vi "cDAQ_VI_Leo_Autotuning.vi"() -> ()   [LabVIEW 2022 SP3]
uses:
  <vilib>/addons/control/pid/autopid.llb/PID autotuning parameters.ctl
  <vilib>/Analysis/baseanly.llb/Mean (DBL).vi
  <vilib>/DAQmx/read.llb/DAQmx Read (Analog 1D Wfm NChan NSamp).vi
  STOP_GLOBAL.vi
  <vilib>/DAQmx/configure/timing.llb/DAQmx Timing (Sample Clock).vi
  <vilib>/addons/control/pid/pid.llb/PID Lead-Lag (DBL).vi
  <vilib>/addons/control/pid/pid.llb/PID Gain Schedule (DBL).vi
  <vilib>/addons/control/pid/pid.llb/PID (DBL).vi
  <vilib>/DAQmx/miscellaneous.llb/DAQmx Fill In Error Info.vi
  <vilib>/Analysis/NI_AALBase.lvlib
  <vilib>/addons/control/pid/NI_PID_pid.lvlib
  <vilib>/ptbypt/NI_PtbyPt.lvlib
  <resource>/objmgr/daqmx.rc
panel:
  out "Inlet Pressure":dynamicdata(graph)
  in  "Channel Array":dbl[](array[slide]) scale=0.0..5.067
  in  "Pressure Scheduling":T1(array[cluster])=[{"PID gains"={"Kc"=7.0, "Ti"=0.001, "Td"=0.0}, "max value"=0.0}] {"max value" format="%.2f"; "PID gains"."Td" format="%#.3g"; "PID gains"."Ti" format="%#.3g"; "PID gains"."Kc" format="%#.3g"}
  out "Runtime Passed?":bool
  in  "RunTime":dbl
  out "Entire Runtime":dbl
  out "Actual Clock Rate":dbl
  out "error out 4":errorcluster
  out "Setpoint profile":dbl
  out "Second Pressure Transducer":cluster{dbl[], dbl[]}(graph)
  out "Line Pressure":dynamicdata(graph)
  out "Servo Voltage Output":cluster{dbl[], dbl[]}(graph)
  in  "Tab Control":T2(tab)
  out "error out 5":errorcluster
  in  "stop":bool
  in  "Needle Valve Control":dbl[](array[slide]) scale=0.0..1.0
  out "Waveform Chart":cluster{"SP":dbl, dbl}(graph)
  out "Output":dbl(slide) scale=0.0..5.067
  out "Process Variable vs Setpoint":cluster{dbl[], dbl[]}[](graph)
  out "error out":errorcluster
  out "element":dbl
  out "MVT Process variable":dbl
  out "MVT Setpoint":dbl
  in  "SP":dbl format="%.2f"
  out "PID gains out":T3={"proportional gain (Kc)"=1.0, "integral time (Ti, min)"=0.01, "derivative time (Td, min)"=0.0} {"derivative time (Td, min)" format="%.3f"; "integral time (Ti, min)" format="%.3f"; "proportional gain (Kc)" format="%.3f"}
  in  "Insert Gain":bool
  out "output":dbl format="%.2f"
  in  "Autotune":bool
  in  "Reinitialize":bool
  in  "Automatic":bool=TRUE
  in  "Replace Gain":bool
  in  "alpha":dbl=nan format="%.2f"
  out "tuned PID gains":T3={"proportional gain (Kc)"=1.0, "integral time (Ti, min)"=0.01, "derivative time (Td, min)"=0.0} {"derivative time (Td, min)" format="%.3f"; "integral time (Ti, min)" format="%.3f"; "proportional gain (Kc)" format="%.3f"}
  out "Voltage Output":dynamicdata(graph)
  in  "autotuning parameters":T4={"type of controller"=0, "relay cycles"=3, "relay amplitude"=1.0, "control specifications"=2, "PV noise level"=0.1} {"PV noise level" format="%.2f"; "control specifications" items=["normal", "fast", "slow"]; "relay amplitude" format="%.2f"; "type of controller" items=["P", "PI", "PID"]}
  out "index out":i32
  in  "MV:":dbl(slide)=30.8641975308642 scale=0.0..5.067 scale format="%.1f"
  out "Waiting \nfor Start":bool=TRUE
  in  "Start VI":bool
  out "Time":dbl
  in  "Gain Schedule":T1(array[cluster])=[{"PID gains"={"Kc"=7.0, "Ti"=0.001, "Td"=0.0}, "max value"=0.0}] {"max value" format="%.2f"; "PID gains"."Td" format="%#.3g"; "PID gains"."Ti" format="%#.3g"; "PID gains"."Kc" format="%#.3g"}
  out "Steps on Servo":dbl[](array[numeric])
  out "Elapsed Time (s) 2":dbl caption="Elapsed Time (s)"
  out "HAS 3 SECONDS PASSED?":bool
  in  "PRESS TO START":bool
  out "All Channel Graph":cluster{dbl[], dbl[]}[](graph)
  out "Thrust":cluster{dbl[], dbl[]}(graph)
  out "Chamber Pressure":cluster{dbl[], dbl[]}(graph)
  out "Supply Pressure":cluster{dbl[], dbl[]}(graph)
  out "MassFlow":cluster{dbl[], dbl[]}(graph)
  out "Temperature":cluster{dbl[], dbl[]}(graph)
  out "error out 3":errorcluster caption="error out"
  out "error out 2":errorcluster
  in  "rate":dbl=1000.0 format="%0.2f"
  in  "number of samples":i32=100
  in  "File Format":string
  in  "File Name Out":string
  in  "Data Collection Folder":path
  out "Temperature":dynamicdata(graph)
  out "Thrust lb":dynamicdata(graph)
  in  "Types of Testing":enum32{"Test Firing", "Cold Flow Rig"}(tab)
  out "Saving Data":bool
  out "Filename Out":path
  in  "Collect Data?":bool=TRUE caption="Enable"
  in  "Collect Data? 2":bool=TRUE caption="Enable"
  out "Saving Data":bool
  out "Filename Out":path
  out "Supply Pressure PSI":dynamicdata(graph)
  out "Vol Flow L/min":dynamicdata(graph)
  out "Chamber Pressure PSI":dynamicdata(graph)
  # "DATA LOGGING INFORMATION"
  # "Control Loop"
  # "ANALOG VOLTAGE OUTPUT"
  # "RESULTS"
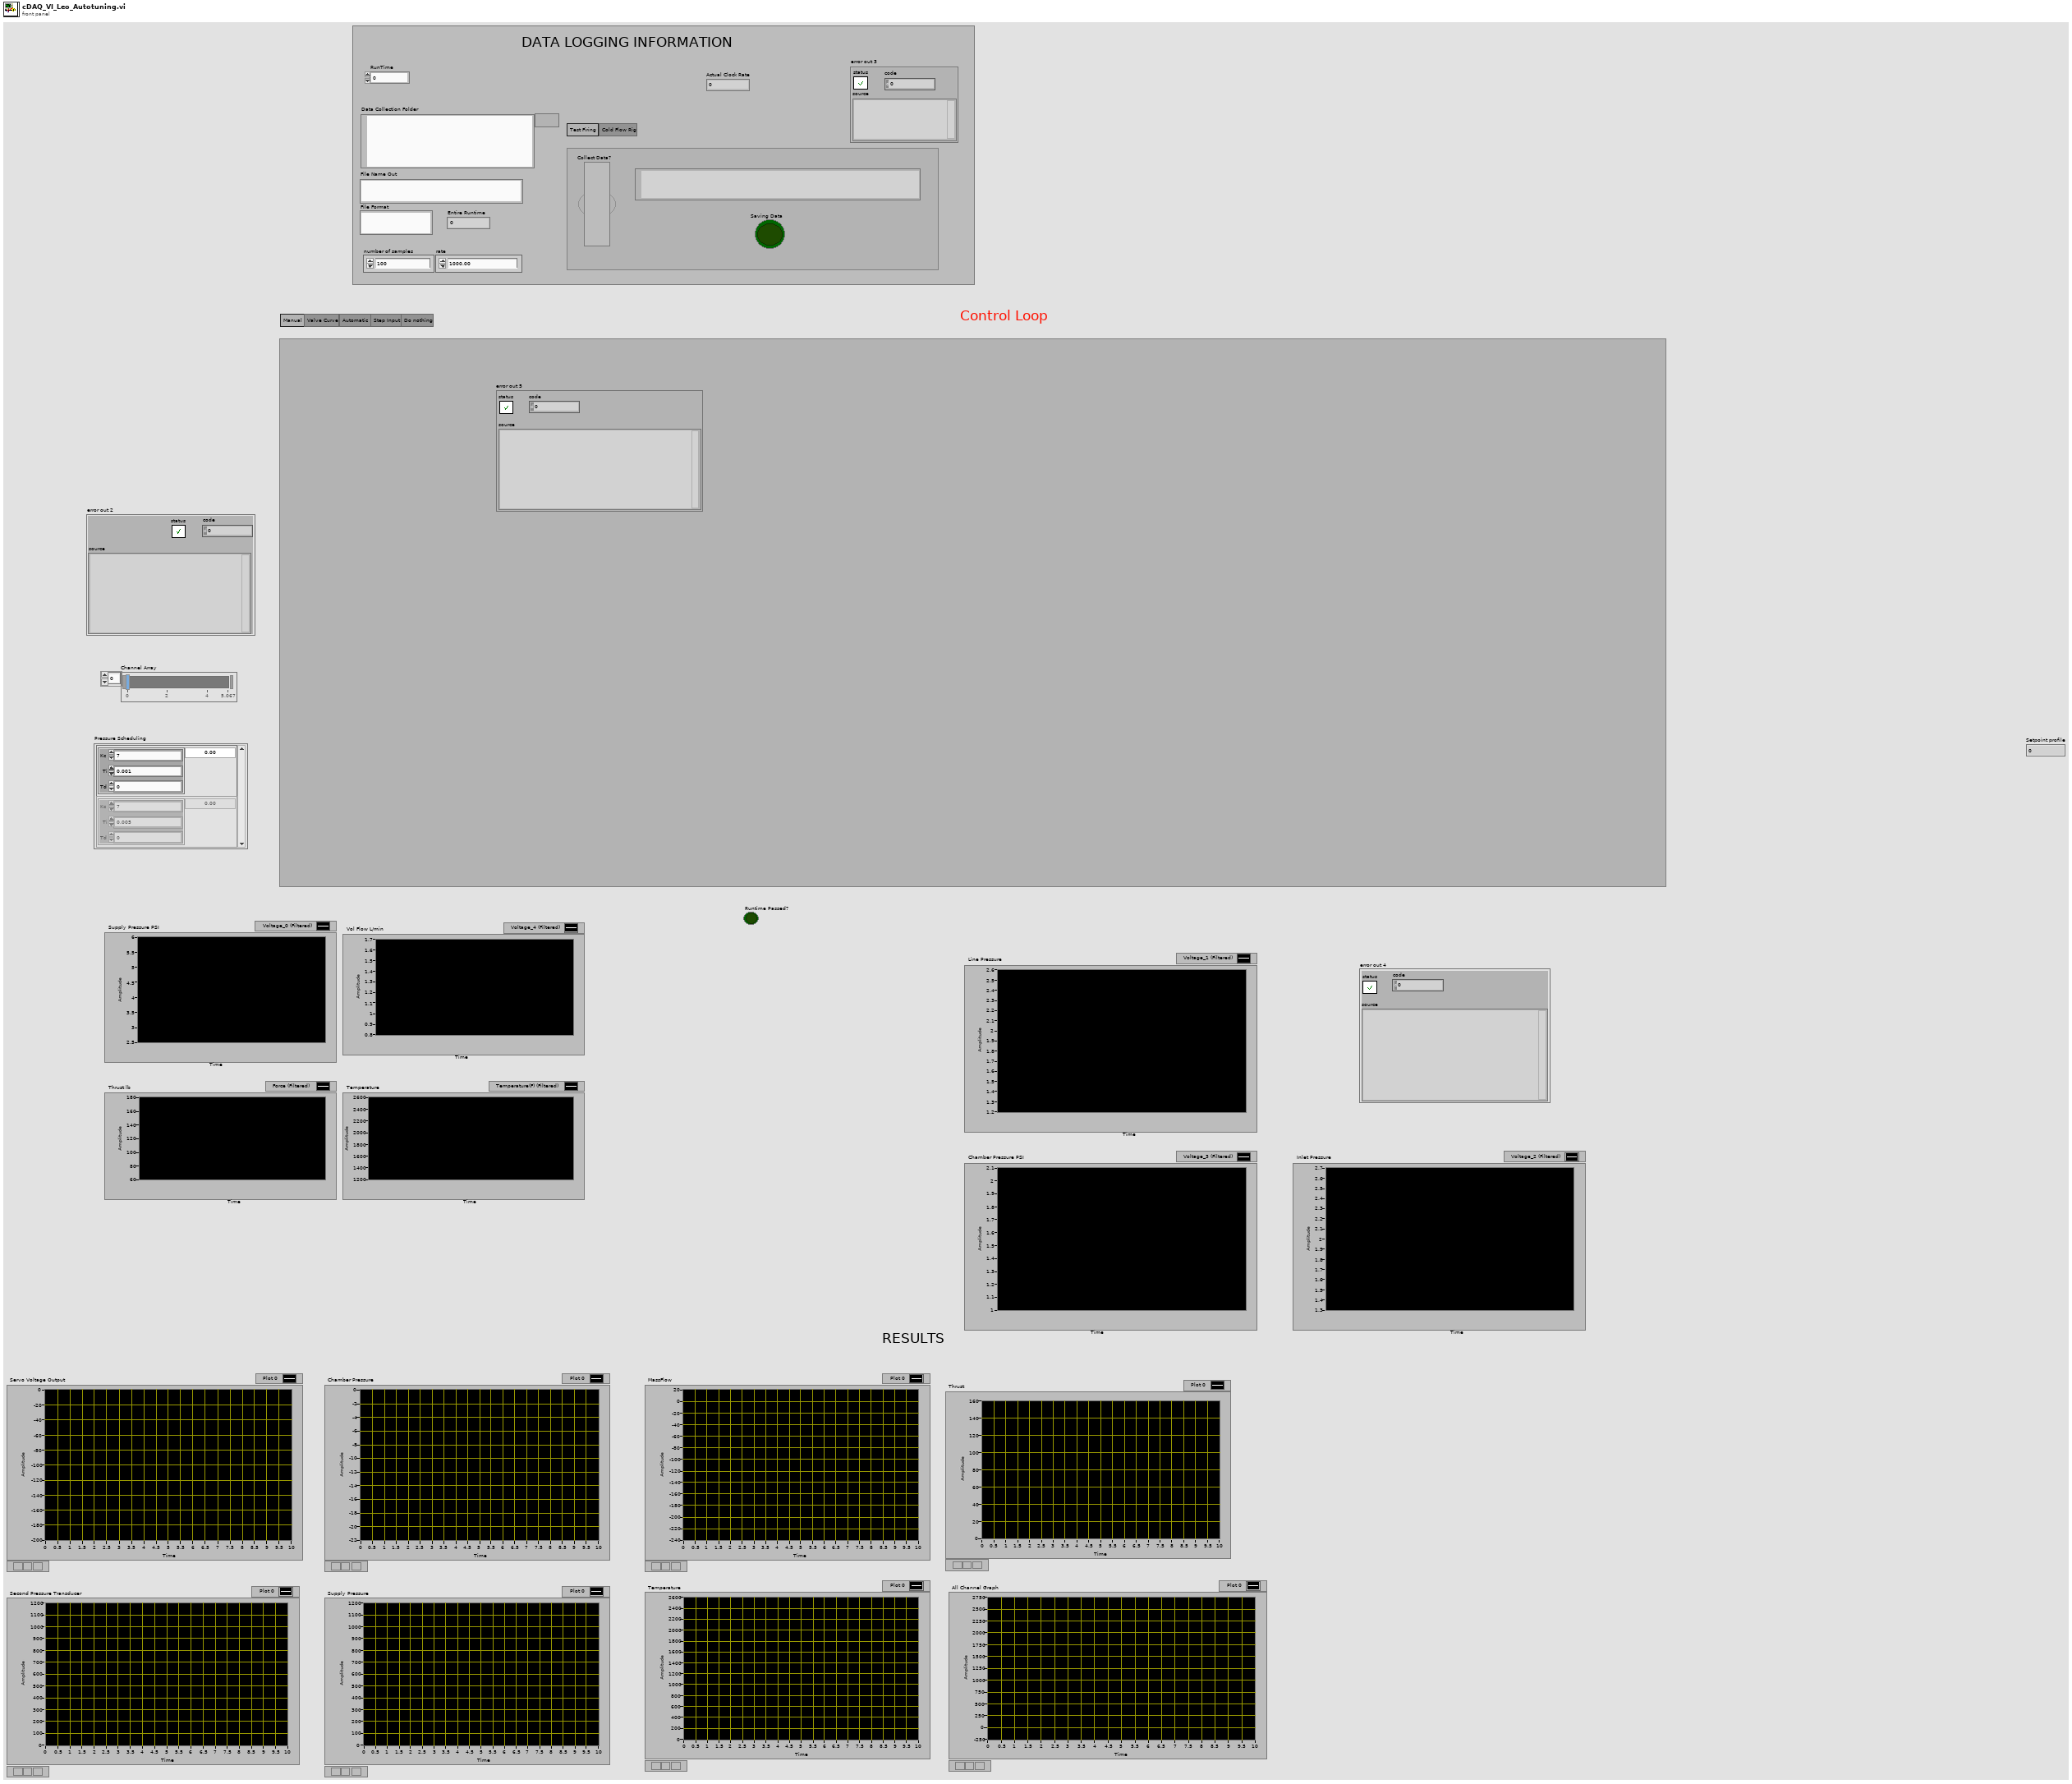
[diagram p1: front panel]
types:
  T1 = cluster{"PID gains":cluster{"Kc":dbl, "Ti":dbl, "Td":dbl}, "max value":dbl}[]
  T2 = enum32{"Manual", "Valve Curve", "Automatic", "Step Input", "Do nothing"}
  T3 = cluster{"proportional gain (Kc)":dbl, "integral time (Ti, min)":dbl, "derivative time (Td, min)":dbl}
  T4 = typedef "PID autotuning parameters.ctl" = cluster{"type of controller":u16, "relay cycles":i32, "relay amplitude":dbl, "control specifications":u16, "PV noise level":dbl}
  T5 = cluster{"Modulus":dbl, "Number of\nComplete Cycles":dbl}
  T6 = cluster{"PID gains":cluster{"Kc":dbl, "Ti":dbl, "Td":dbl}, "max value":dbl}
  T7 = cluster{"Tuned PID gains":cluster{"proportional gain (Kc)":dbl, "integral time (Ti, min)":dbl, "derivative time (Td, min)":dbl}, "MVT Process Variable":dbl}
  T8 = cluster{"Tuned PID gains":cluster{"proportional gain (Kc)":dbl, "integral time (Ti, min)":dbl, "derivative time (Td, min)":dbl}, "max value":dbl}
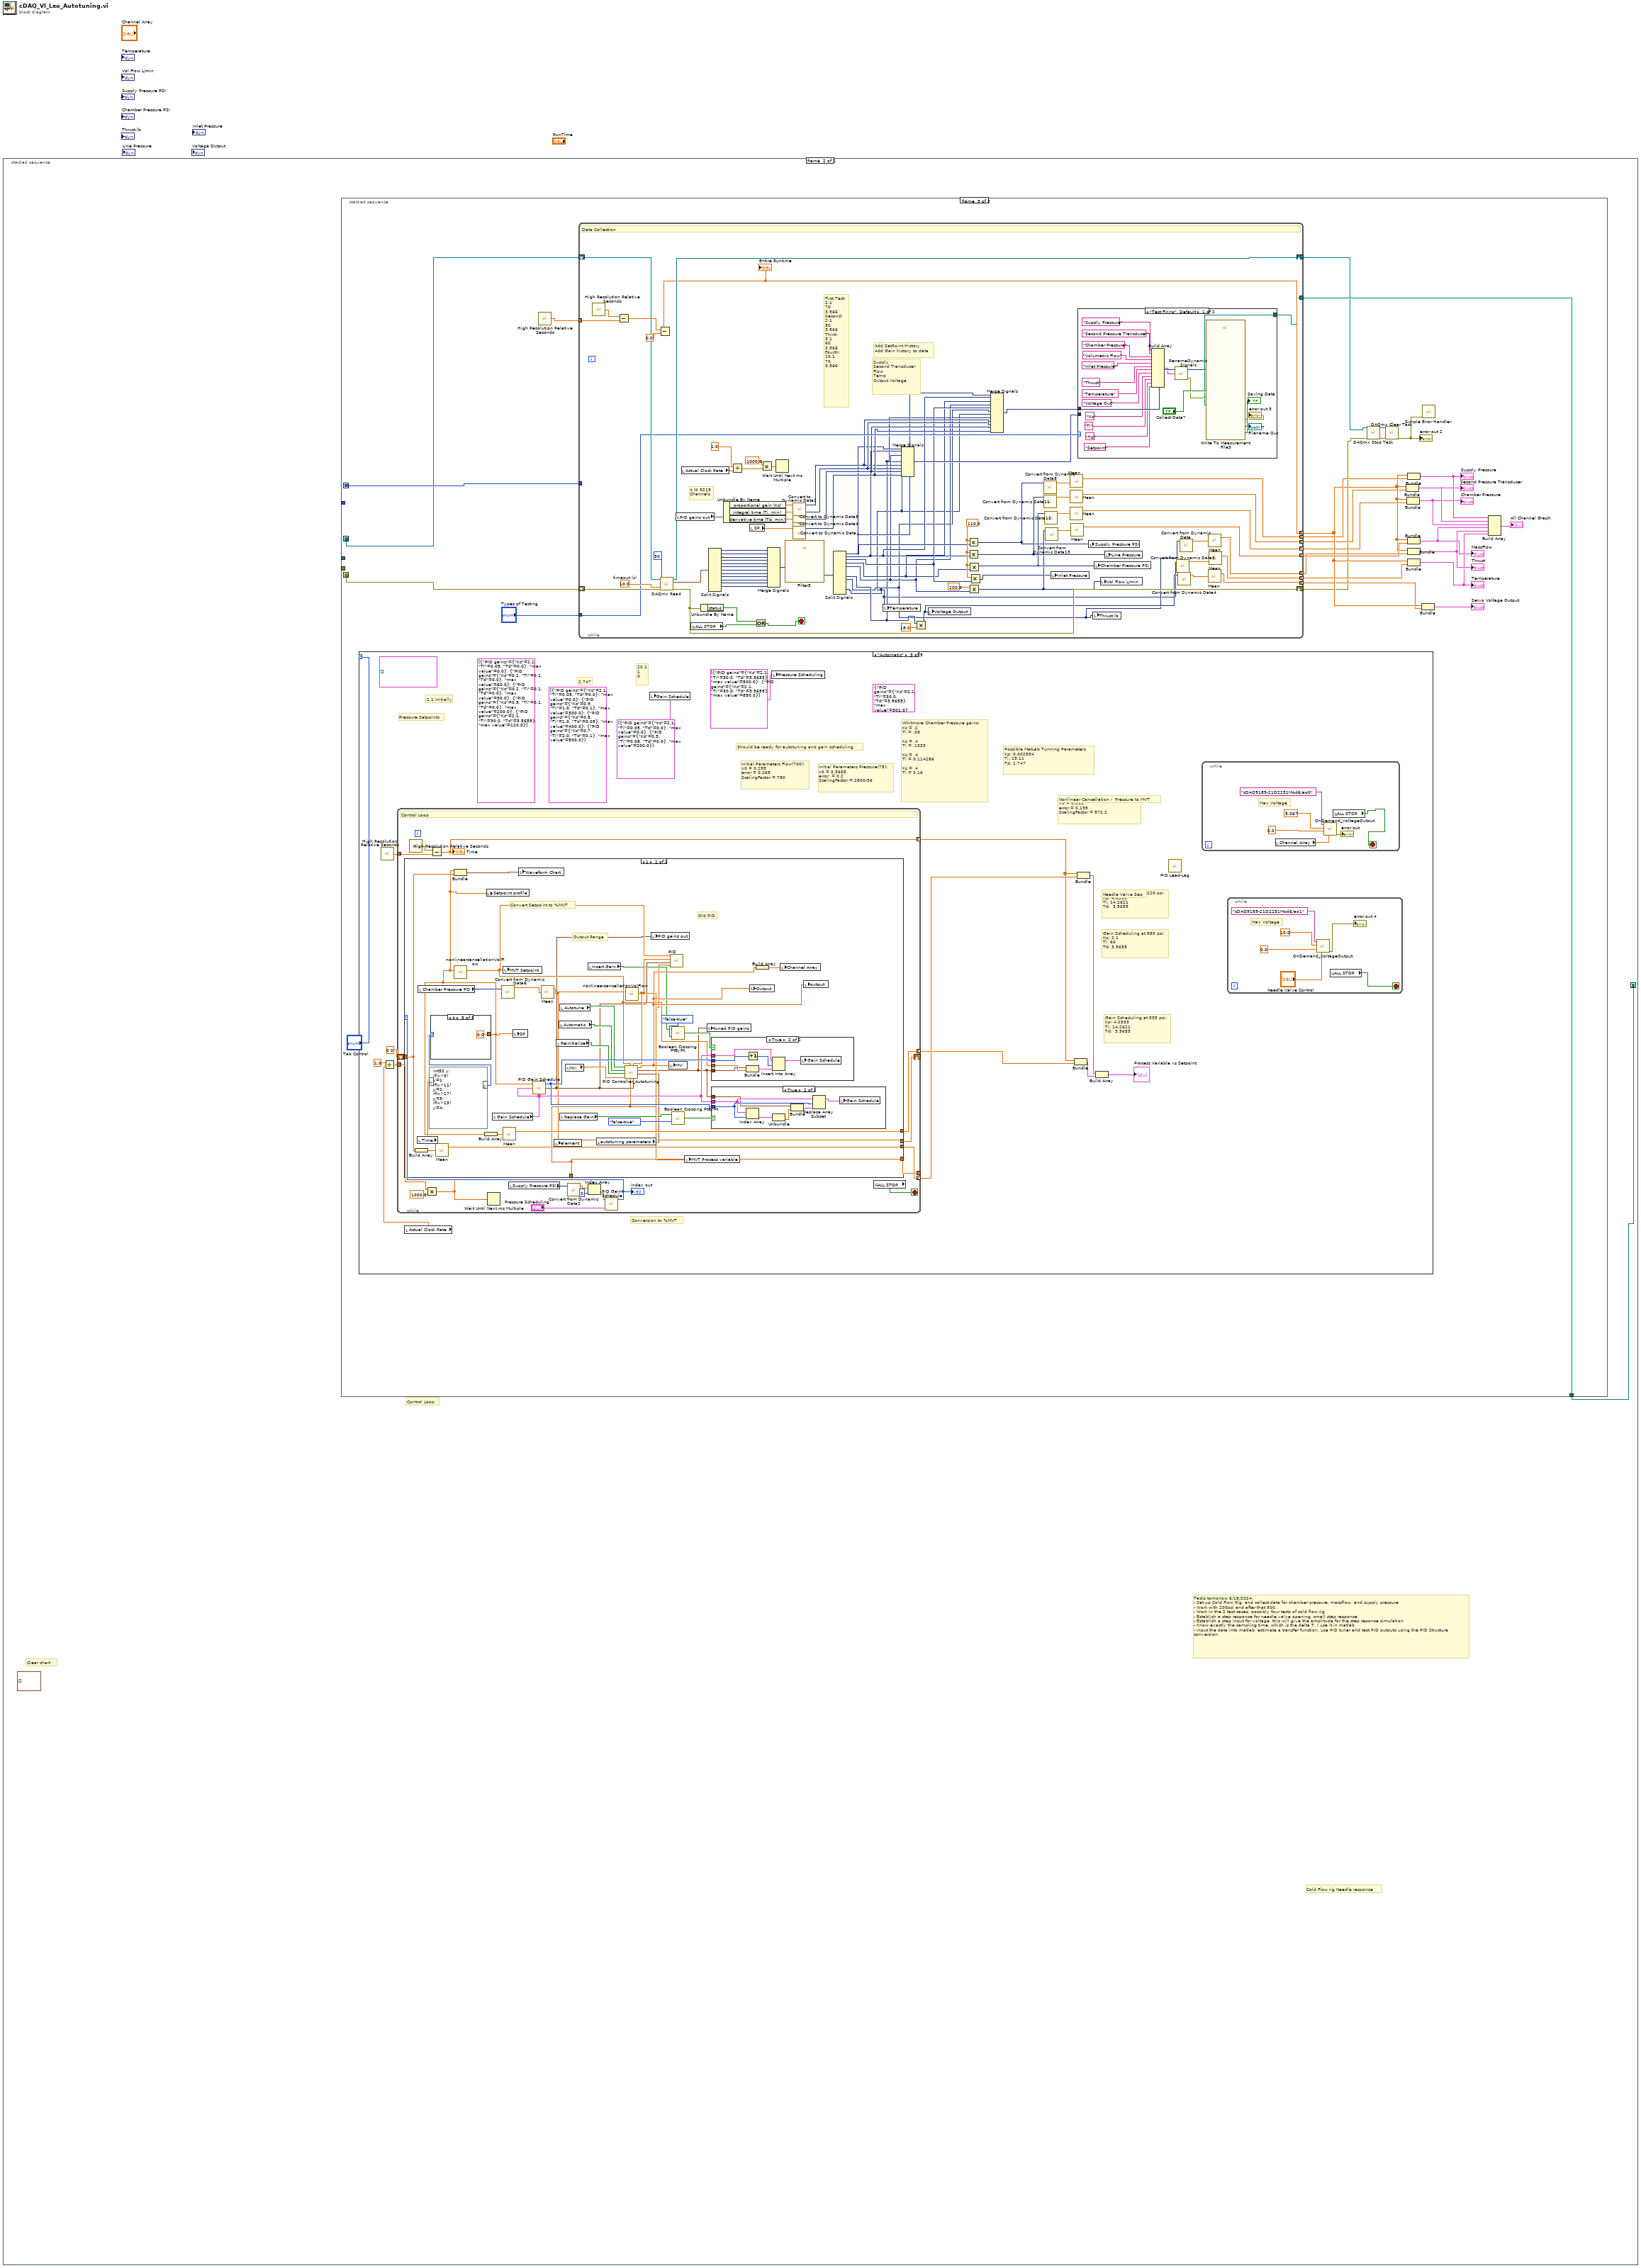
[diagram p0: block diagram]
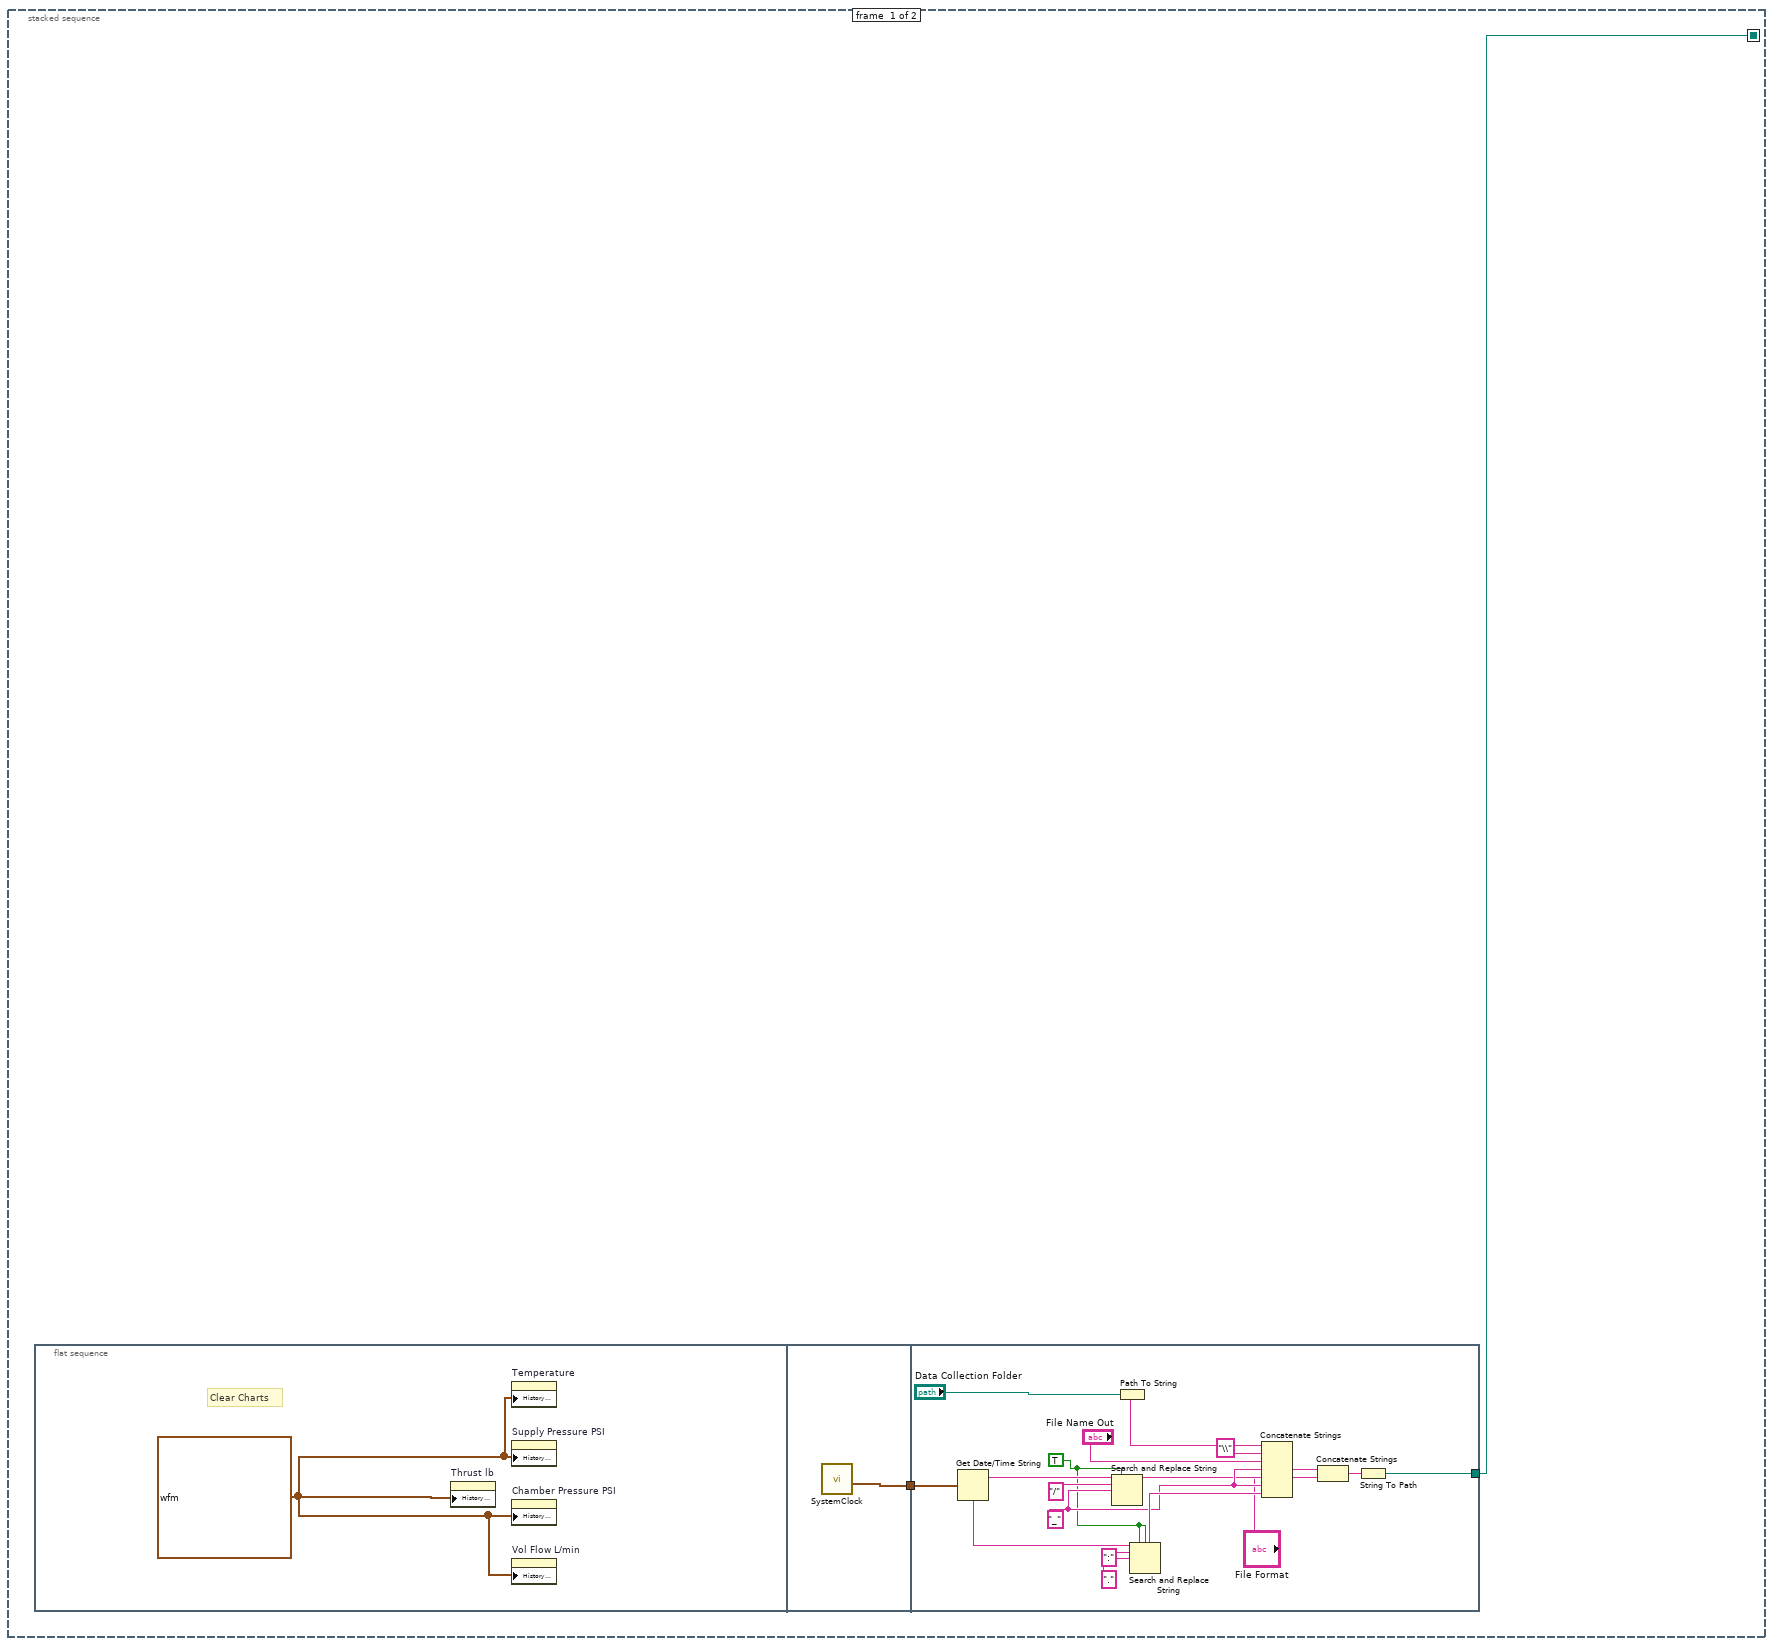
[diagram p2: hidden frame]
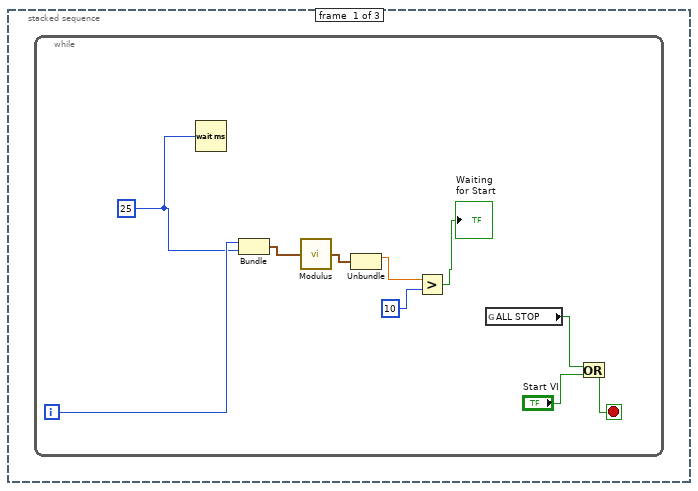
[diagram p3: hidden frame]
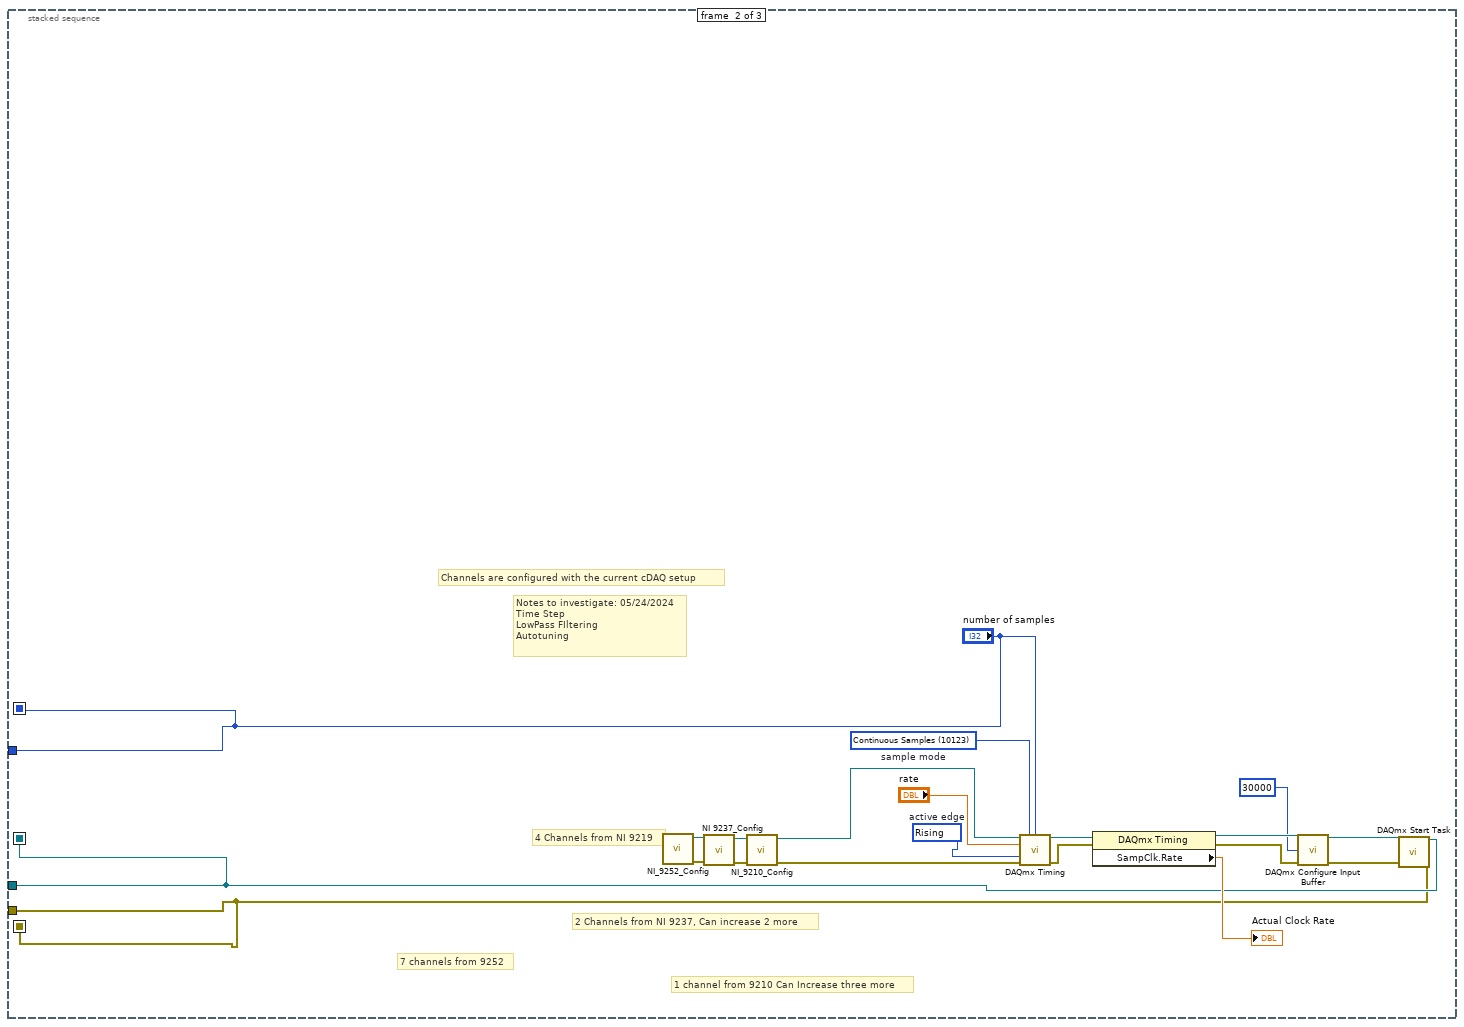
[diagram p4: hidden frame]
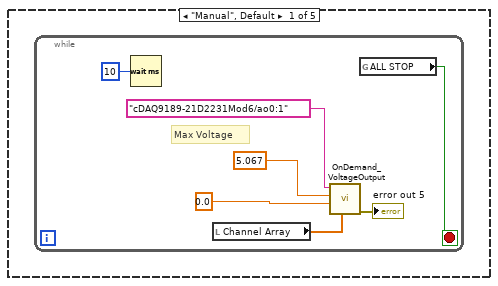
[diagram p5: hidden frame]
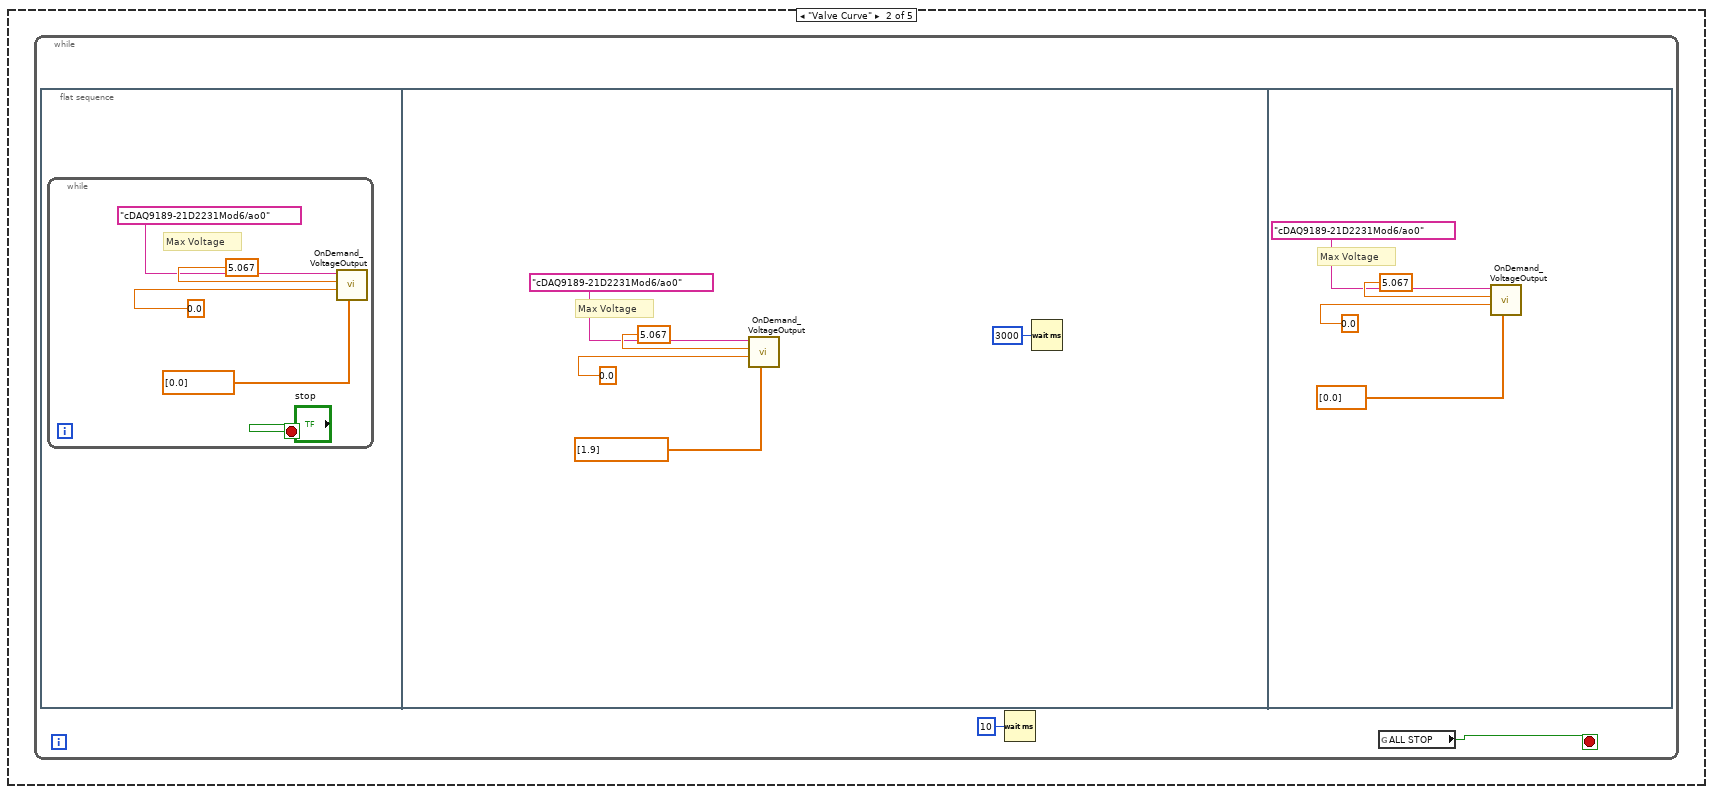
[diagram p6: hidden frame]
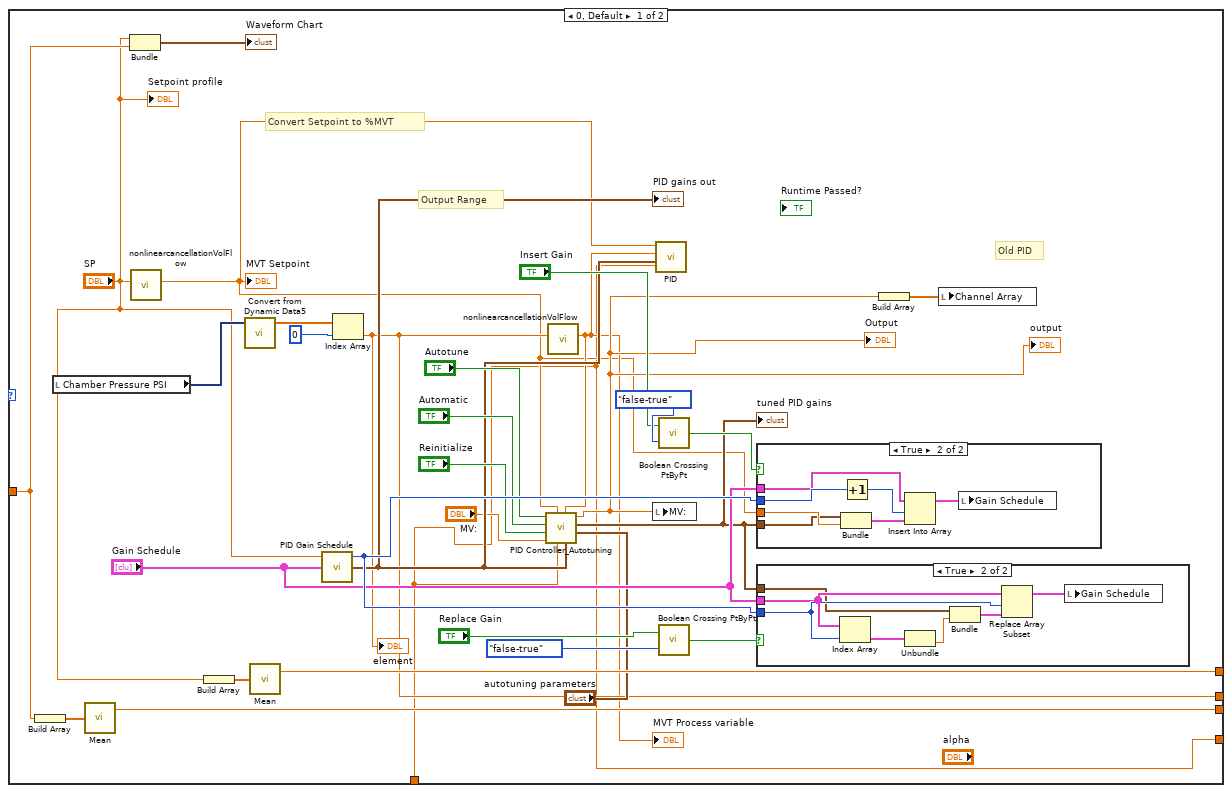
[diagram p7: hidden frame]
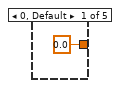
[diagram p10: hidden frame]
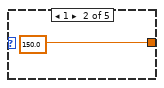
[diagram p11: hidden frame]
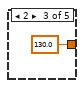
[diagram p12: hidden frame]
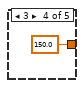
[diagram p13: hidden frame]
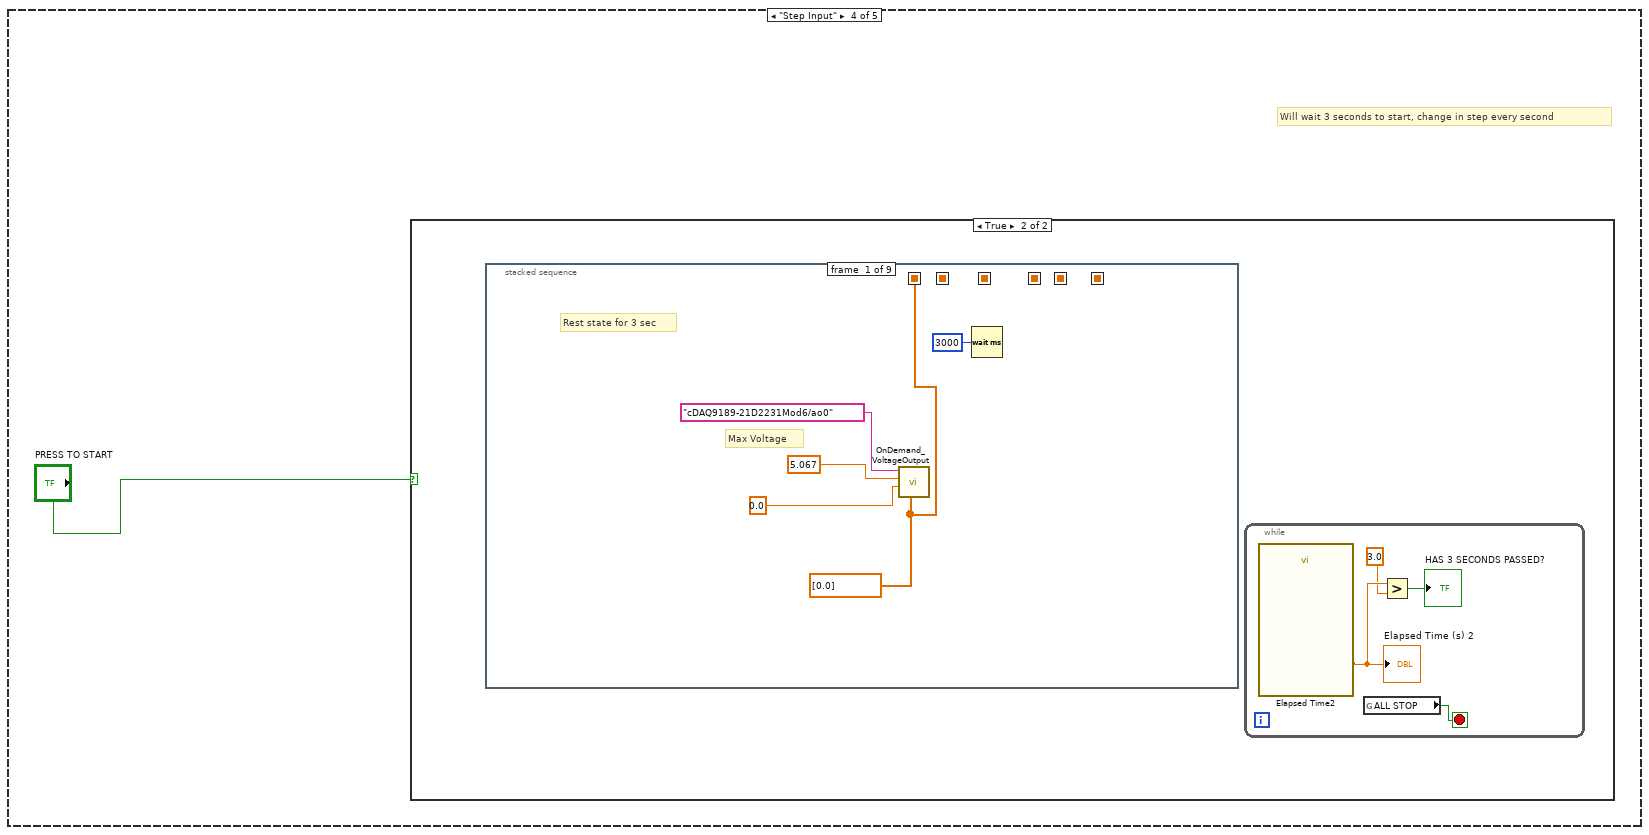
[diagram p16: hidden frame]
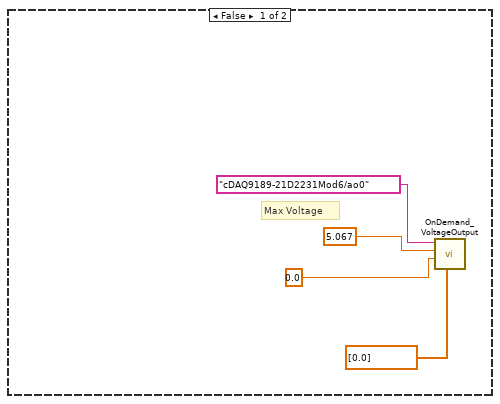
[diagram p17: hidden frame]
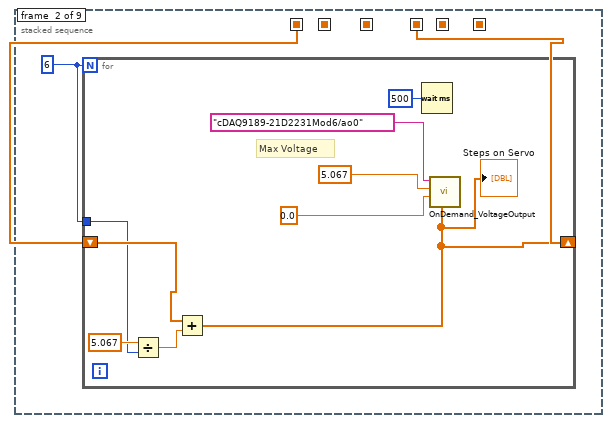
[diagram p18: hidden frame]
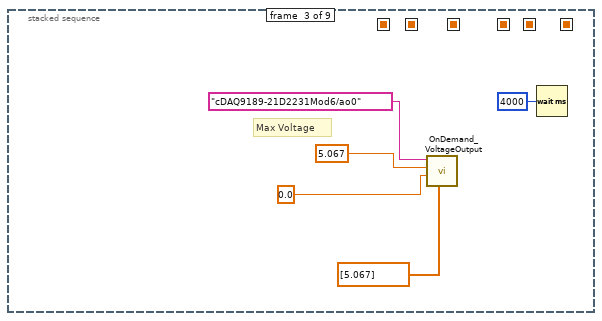
[diagram p19: hidden frame]
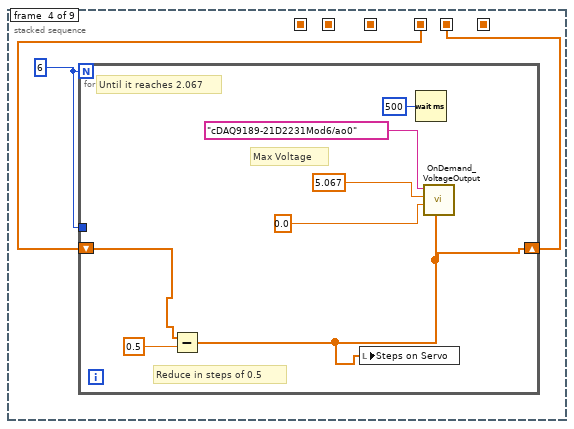
[diagram p20: hidden frame]
diagram:
  n1 = stacked-sequence {
    seq-local: [w1 _] -> [_ w23]
    frame #0 {
      n2 = flat-sequence {
        tunnel: [w4] -> w2
        tunnel: w2 -> [w11]
        tunnel: [w10] -> w1
        frame #0 {
          w3 = waveform(dbl)[] [{"t0"=timestamp(0 s since 1904-01-01), "dt"=1.0, "Y"=[]}]
          # "Clear Charts"
          n3 = property on="Thrust lb" class="WFChart (strict)"("History Data"=w3) -> ()  [unwired: 2 in, 2 out]
          n4 = property on="Temperature" class="WFChart (strict)"("History Data"=w3) -> ()  [unwired: 2 in, 2 out]
          n5 = property on="Supply Pressure PSI" class="WFChart (strict)"("History Data"=w3) -> ()  [unwired: 2 in, 2 out]
          n6 = property on="Chamber Pressure PSI" class="WFChart (strict)"("History Data"=w3) -> ()  [unwired: 2 in, 2 out]
          n7 = property on="Vol Flow L/min" class="WFChart (strict)"("History Data"=w3) -> ()  [unwired: 2 in, 2 out]
        }
        frame #1 {
          n8 = call "SystemClock.vi"() -> ("LabVIEW Time Stamp"=w4:timestamp)  [unwired: 9 in, 2 out]
        }
        frame #2 {
          w6 = TRUE ("replace all? (F)")
          w19 = "_" ("string")
          n9 = Get Date/Time String(seconds (now)=w11) -> (date string=w13:string, time string=w16:string)  [unwired: 2 in]
          n10 = Search and Replace String(replace all?=w6, input string=w13, search string="/", replace string=w19) -> (result string=w15:string)  [unwired: 4 in, 3 out]
          n11 = Path To String(path="Data Collection Folder") -> (string=w8:string)
          n12 = Search and Replace String(replace all?=w6, case sensitive?=w6, input string=w16, search string=":", replace string="." ("replace string (\"\")")) -> (result string=w20:string)  [unwired: 3 in, 3 out]
          n13 = Concatenate Strings(w8, "\\" ("string"), "File Name Out", w19, w15, w19, w20) -> (w21:string)
          n14 = Concatenate Strings(w21, "File Format") -> (w22:string)
          n15 = String To Path(string=w22) -> (path=w10:path)
        }
      }
    }
    frame #1 {
      (unwired) cluster{"setpoint":dbl, dbl}[] [] ("History Data")
      # "Cold Flow rig Needle response"
      # "Tasks tomorrow 6/15/2024:\n- Set up Cold Flow Rig, and collect data for chamber pressure, massflow, and supply pressure\n- Work with 200psi and after that 500.\n- Work in the 2 test cases, possibly four tests of cold flow rig\n- Establish a step response for needle valve opening, small step response\n- Establish a step input for voltage, this will give the amplitude for the step reponse simulation\n- Know exactly the sampling time, which is the delta T, I use it in matlab\n- Input the data into matlab, estimate a transfer function, use PID tuner and test PID outputs using the PID Structure\nconversion."
      # "Control Loop"
      # "Clear chart"
      n16 = stacked-sequence {
        seq-local: [_ "number of samples" _] -> [_ _ w63]
        seq-local: [_ w39 _] -> [_ _ w62]
        seq-local: [_ w38 _] -> [_ _ w61]
        tunnel: w23 -> [_ _ w59]
        tunnel: [_ w39 _] -> _
        tunnel: [_ w38 _] -> _
        tunnel: [_ "number of samples" _] -> _
        frame #0 {
          n17 = while {
            i -> [w33]
            stop <- w25 stop-if-true
            w24 = u32 25 ("milliseconds to wait")
            n18 = Wait (ms)(milliseconds to wait=w24) -> ()  [unwired: 1 out]
            n19 = Bundle(w33, "milliseconds to wait"=w24) -> (w32:cluster{i32, "milliseconds to wait":u32})  [unwired: 1 in]
            n20 = call "Modulus.vi"("Input"=w32) -> ("Output"=w31:T5)
            n21 = Unbundle(w31) -> ("Modulus"=w30:dbl)  [unwired: 1 out]
            n22 = Greater?(x=w30, y=u32 10 ("milliseconds to wait")) -> (0:→"Waiting \nfor Start":bool)
            n23 = global read "STOP_GLOBAL.vi" "ALL STOP"() -> (w27:bool)
            n24 = Or(x=w27, y="Start VI") -> (x .or. y?=w25:bool)
          }
        }
        frame #1 {
          w42 = 10123 items=["Finite Samples"=10178, "Continuous Samples"=10123, "Hardware Timed Single Point"=12522]  # sample mode
          w41 = 10280 items=["Rising"=10280, "Falling"=10171]  # active edge
          # "Notes to investigate: 05/24/2024\nTime Step\nLowPass FIltering\nAutotuning"
          # "Channels are configured with the current cDAQ setup"
          # "7 channels from 9252"
          # "1 channel from 9210 Can Increase three more"
          # "2 Channels from NI 9237, Can increase 2 more"
          # "4 Channels from NI 9219"
          n25 = call "NI_9252_Config.vi"() -> ("error out"=w36:errorcluster, "task out"=w37:refnum<k21>)  [unwired: 10 in]
          n26 = call "NI 9237_Config.vi"("error in"=w36, "task in"=w37) -> ("error out"=w45:errorcluster, "task out"=w44:refnum<k21>)  [unwired: 8 in]
          n27 = call "NI_9210_Config.vi"("error in"=w45, "task in"=w44) -> ("error out"=w34:errorcluster, "task out"=w35:refnum<k21>)  [unwired: 8 in]
          n28 = call-poly <vilib>:"DAQmx Timing.vi"("task/channels in"=w35, "sample mode"=w42, "samples per channel"="number of samples", "rate"="rate", "active edge"=w41, "error in"=w34) -> ("task out"=w47:refnum<k21>, "error out"=w48:errorcluster)  [unwired: 8 in]
          n29 = property class="DAQmx Timing"(reference=w47, error in=w48) -> (reference out=w49:refnum<k21>, error out=w50:errorcluster, "SampClk.Rate"=→"Actual Clock Rate":dbl)
          n30 = call <vilib>:"DAQmx Configure Input Buffer.vi"("task/channels in"=w49, "buffer size (in samples per channel)"=u32 30000, "error in"=w50) -> ("task out"=w52:refnum<k21>, "error out"=w51:errorcluster)  [unwired: 11 in]
          n31 = call <vilib>:"DAQmx Start Task.vi"("task/channels in"=w52, "error in"=w51) -> ("task out"=w39:refnum<k21>, "error out"=w38:errorcluster)  [unwired: 12 in]
        }
        frame #2 {
          n32 = case shown="\"Automatic\"" "Tab Control" {
            frame "Manual", Default {
              n33 = while {
                stop <- w88 stop-if-true
                # "Max Voltage"
                n34 = Wait (ms)(milliseconds to wait=u32 10) -> ()  [unwired: 1 out]
                n35 = local read "Channel Array"() -> (w84:dbl[])
                n36 = call "OnDemand_VoltageOutput.vi"("Channel Array"=w84, "minimum voltage"=0.0, "maximum voltage"=5.067, "physical channels"="cDAQ9189-21D2231Mod6/ao0:1") -> ("error out"=→"error out 5":errorcluster)  [unwired: 5 in, 2 out]
                n37 = global read "STOP_GLOBAL.vi" "ALL STOP"() -> (w88:bool)
              }
            }
            frame "Valve Curve" {
              n38 = while {
                stop <- w89 stop-if-true
                n39 = flat-sequence {
                  frame #0 {
                    n40 = while {
                      stop <- "stop" stop-if-true
                      # "Max Voltage"
                      n41 = call "OnDemand_VoltageOutput.vi"("Channel Array"=dbl[] [0.0], "minimum voltage"=0.0, "maximum voltage"=5.067, "physical channels"="cDAQ9189-21D2231Mod6/ao0") -> ()  [unwired: 5 in, 3 out]
                    }
                  }
                  frame #1 {
                    # "Max Voltage"
                    n42 = call "OnDemand_VoltageOutput.vi"("Channel Array"=dbl[] [1.9], "minimum voltage"=0.0, "maximum voltage"=5.067, "physical channels"="cDAQ9189-21D2231Mod6/ao0") -> ()  [unwired: 5 in, 3 out]
                    n43 = Wait (ms)(milliseconds to wait=u32 3000) -> ()  [unwired: 1 out]
                  }
                  frame #2 {
                    # "Max Voltage"
                    n44 = call "OnDemand_VoltageOutput.vi"("Channel Array"=dbl[] [0.0], "minimum voltage"=0.0, "maximum voltage"=5.067, "physical channels"="cDAQ9189-21D2231Mod6/ao0") -> ()  [unwired: 5 in, 3 out]
                  }
                }
                n45 = Wait (ms)(milliseconds to wait=u32 10) -> ()  [unwired: 1 out]
                n46 = global read "STOP_GLOBAL.vi" "ALL STOP"() -> (w89:bool)
              }
            }
            frame "Automatic" {
              (unwired) T6 {"PID gains"={"Kc"=2.1, "Ti"=30.0, "Td"=3.5655}, "max value"=301.0} ("gain schedule")
              (unwired) T1 [{"PID gains"={"Kc"=2.1, "Ti"=0.05, "Td"=0.0}, "max value"=0.0}, {"PID gains"={"Kc"=0.9, "Ti"=1.0, "Td"=0.1}, "max value"=300.0}, {"PID gains"={"Kc"=0.8, "Ti"=1.0, "Td"=0.09}, "max value"=400.0}, {"PID gains"={"Kc"=0.7, "Ti"=2.0, "Td"=0.1}, "max value"=500.0}]
              (unwired) T1 [{"PID gains"={"Kc"=2.1, "Ti"=0.05, "Td"=0.0}, "max value"=0.0}, {"PID gains"={"Kc"=0.1, "Ti"=0.1, "Td"=0.0}, "max value"=60.0}, {"PID gains"={"Kc"=0.2, "Ti"=0.1, "Td"=0.0}, "max value"=90.0}, {"PID gains"={"Kc"=0.5, "Ti"=0.1, "Td"=0.0}, "max value"=200.0}, {"PID gains"={"Kc"=2.1, "Ti"=30.0, "Td"=3.5655}, "max value"=120.0}] ("PID gain schedule 2")
              (unwired) T1 [] ("PID gain schedule 2")
              # "Whitmore Chamber Pressure gains:\nKc = .2\nTi = .08\n\nKc = .4\nTi = .1333\n\nKc = .4\nTi = 0.114286\n\nKc = .4\nTi = 0.16"
              # "Conversion to %MVT"
              # "Pressure Setpoints"
              # "Initial Parameters Pressure(75):\nx0 = 0.3665\nerror  = 0.2\nScalingFactor = 2800/36"
              # "Initial Parameters Flow(700):\nx0 = 0.295\nerror = 0.265\nScalingFactor = 780"
              # "2.1 Initially"
              # "20.1\n1\n0"
              # "2.747"
              # "Should be ready for autotuning and gain scheduling"
              # "Possible parameters for 800 SLM:\nx0 = 0.315\nerror = 0.195\nScalingFactor = 972.2"
              # "Nonlinear Cancellation -  Pressure to MVT"
              # "Possible MatLab Tunning Parameters\nKp: 0.002894\nTi: 25.11\nTd: 2.747"
              # "Gain Scheduling at 335 psi:\nKp: 4.0333\nTi: 14.2621\nTd:  3.5655"
              # "Gain Scheduling at 855 psi:\nKp: 2.1\nTi: 60\nTd: 3.5655"
              # "Gain Scheduling at 220 psi:\nKp: 4.0333\nTi: 14.2621\nTd:  3.5655"
              # "Needle Valve Seq"
              n47 = call <vilib>:"High Resolution Relative Seconds.vi"() -> ("relative seconds"=w112:dbl)
              n48 = local read "Actual Clock Rate"() -> (w111:dbl)
              n49 = Divide(x=1.0, y=w111) -> (x/y=w109:dbl)
              n50 = while {
                shift-right: [w141] -> _
                shift-left: 0.0 -> [w139]
                tunnel: [w140] -> w115 mode=indexing
                tunnel: [w147] -> w108 mode=indexing
                tunnel: [w146] -> w107 mode=indexing
                tunnel: w112 -> [w145]
                tunnel: [w142] -> _
                tunnel: w109 -> [w131]
                stop <- w143 stop-if-true
                # "Control Loop"
                n51 = call <vilib>:"High Resolution Relative Seconds.vi"() -> ("relative seconds"=w144:dbl)
                n52 = Multiply(x=w131, y=1000.0) -> (x*y=w130:dbl)
                n53 = Subtract(x=w144, y=w145) -> (x-y=w140:dbl)
                "Time" <- w140
                n54 = Wait Until Next ms Multiple(millisecond multiple=w130) -> ()  [unwired: 1 out]
                n55 = local read "Supply Pressure PSI"() -> (w138:dynamicdata)
                n56 = call "Convert from Dynamic Data2"("Dynamic Data Type"=w138) -> ("Array"=w137:dbl[])  [unwired: 3 in]
                n57 = Index Array(array=w137, index=0) -> (element=w136:dbl)
                n58 = call-poly <vilib>:"PID Gain Schedule.vi"("PID gain schedule"="Pressure Scheduling", "gain scheduling value"=w136) -> ("index out"=w133:i32)  [unwired: 2 in, 1 out]
                "index out" <- w133
                n59 = case shown="1" w133 {
                  tunnel: [w178 w224] -> w147
                  tunnel: [w177 w223] -> w146
                  tunnel: [w148 w198] -> w142
                  tunnel: [w156 w199] -> w141
                  tunnel: w139 -> [w153 w214]
                  tunnel: w130 -> [w148 w198]
                  frame 0, Default {
                    # "Old PID"
                    # "Convert Setpoint to %MVT"
                    # "Output Range"
                    n60 = Build Array(w153) -> (w152:dbl[])
                    n61 = local read "Chamber Pressure PSI"() -> (w164:dynamicdata)
                    n62 = call-poly <vilib>:"Mean.vi"("X"=w152) -> ("mean"=w178:dbl)  [unwired: 1 out]
                    n63 = Bundle("SP"="SP", w153) -> (→"Waveform Chart":cluster{"SP":dbl, dbl})  [unwired: 1 in]
                    n64 = call "nonlinearcancellationVolFlow.vi"("input variable"="SP") -> ("MVT Process Variable"=w151:dbl)  [unwired: 10 in]
                    "MVT Setpoint" <- w151
                    n65 = Build Array("SP") -> (w175:dbl[])
                    n66 = call "Convert from Dynamic Data5"("Dynamic Data Type"=w164) -> ("Array"=w174:dbl[])  [unwired: 3 in]
                    n67 = call-poly <vilib>:"Mean.vi"("X"=w175) -> ("mean"=w177:dbl)  [unwired: 1 out]
                    n68 = call-poly <vilib>:"PID Gain Schedule.vi"("PID gain schedule"="Gain Schedule", "gain scheduling value"="SP") -> ("PID gains out"=w159:T3, "index out"=w167:i32)  [unwired: 2 in]
                    "PID gains out" <- w159
                    n69 = Index Array(array=w174, index=0) -> (element=w156:dbl)
                    "element" <- w156
                    n70 = call "nonlinearcancellationVolFlow.vi"("input variable"=w156) -> ("MVT Process Variable"=w154:dbl)  [unwired: 10 in]
                    "MVT Process variable" <- w154
                    n71 = call "PID Controller_Autotuning.vi"("autotuning parameters"="autotuning parameters", "PID gains in"=w159, "process variable"=w154, "dt (s)"=w148, "setpoint"=w151, "manipulated variable"="MV:", "Reinitialize"="Reinitialize", "Automatic"="Automatic", "Autotune"="Autotune") -> ("Tuned PID gains"=w155:T3, "output"=w157:dbl)  [unwired: 1 in]
                    "tuned PID gains" <- w155
                    "Output" <- w157
                    "output" <- w157
                    n72 = local write "MV:"(w157) -> ()
                    n73 = call-poly <vilib>:"PID.vi"("dt (s)"=w148, "PID gains"=w159, "process variable"=w154, "setpoint"=w151) -> ()  [unwired: 6 in, 2 out]
                    n74 = call <vilib>:"Boolean Crossing PtByPt.vi"("direction"=enum16{"either", "false-true", "true-false"}."false-true", "input"="Insert Gain") -> ("crossing"=w172:bool)  [unwired: 1 in]
                    n75 = call <vilib>:"Boolean Crossing PtByPt.vi"("direction"=enum16{"either", "false-true", "true-false"}."false-true", "input"="Replace Gain") -> ("crossing"=w168:bool)  [unwired: 1 in]
                    n76 = case shown="True" w172 {
                      tunnel: w167 -> [_ w192]
                      tunnel: "Gain Schedule" -> [_ w190]
                      tunnel: w151 -> [_ w189]
                      tunnel: w155 -> [_ w187]
                      frame False {
                      }
                      frame True {
                        n77 = Bundle("Tuned PID gains"=w187, "MVT Process Variable"=w189) -> (w186:T7)  [unwired: 1 in]
                        n78 = Increment(x=w192) -> (x+1=w191:i32)
                        n79 = Insert Into Array(array=w190, index=w191, new element=w186) -> (w188:T1)
                        n80 = local write "Gain Schedule"(w188) -> ()
                      }
                    }
                    n81 = case shown="True" w168 {
                      tunnel: w167 -> [_ w183]
                      tunnel: "Gain Schedule" -> [_ w182]
                      tunnel: w155 -> [_ w180]
                      frame False {
                      }
                      frame True {
                        n82 = Index Array(array=w182, index=w183) -> (element=w185:T6)
                        n83 = Unbundle(w185) -> ("max value"=w184:dbl)  [unwired: 1 out]
                        n84 = Bundle("Tuned PID gains"=w180, "max value"=w184) -> (w179:T8)  [unwired: 1 in]
                        n85 = Replace Array Subset(array=w182, new element=w179, index=w183) -> (w181:T1)
                        n86 = local write "Gain Schedule"(w181) -> ()
                      }
                    }
                    n87 = Build Array(w157) -> (w149:dbl[])
                    n88 = local write "Channel Array"(w149) -> ()
                    "Setpoint profile" <- "SP"
                  }
                  frame 1 {
                    # "Old PID"
                    # "Convert Setpoint to %MVT"
                    # "Output Range"
                    n89 = Build Array(w214) -> (w213:dbl[])
                    n90 = local read "Time"() -> (w196:dbl)
                    n91 = local read "Chamber Pressure PSI"() -> (w216:dynamicdata)
                    n92 = formula code="int32 y;\nif(x>3)\ny=1;\nif(x>11)\ny=2;\nif(x>17)\ny=3;\nif(x>23)\ny=4;"("x"=w196) -> ("y"=w197:i32)
                    n93 = case shown="4" w197 {
                      tunnel: [0.0 ("SP") 150.0 ("SP") 130.0 ("SP") 150.0 ("SP") 0.0 ("SP")] -> w194
                      frame 0, Default {
                      }
                      frame 1 {
                      }
                      frame 2 {
                      }
                      frame 3 {
                      }
                      frame 4 {
                      }
                    }
                    n94 = call-poly <vilib>:"Mean.vi"("X"=w213) -> ("mean"=w224:dbl)  [unwired: 1 out]
                    n95 = Bundle("SP"=w194, w214) -> (w206:cluster{"SP":dbl, dbl})  [unwired: 1 in]
                    n96 = call "nonlinearcancellationVolFlow.vi"("input variable"=w194) -> ("MVT Process Variable"=w204:dbl)  [unwired: 10 in]
                    n97 = Build Array(w194) -> (w222:dbl[])
                    n98 = local write "Setpoint profile"(w194) -> ()
                    n99 = local read "Gain Schedule"() -> (w212:T1)
                    n100 = call "Convert from Dynamic Data6"("Dynamic Data Type"=w216) -> ("Array"=w195:dbl[])  [unwired: 3 in]
                    n101 = local write "MVT Setpoint"(w204) -> ()
                    n102 = call-poly <vilib>:"Mean.vi"("X"=w222) -> ("mean"=w223:dbl)  [unwired: 1 out]
                    n103 = local write "SP"(w194) -> ()
                    n104 = local write "Waveform Chart"(w206) -> ()
                    n105 = call-poly <vilib>:"PID Gain Schedule.vi"("PID gain schedule"=w212, "gain scheduling value"=w194) -> ("PID gains out"=w203:T3, "index out"=w217:i32)  [unwired: 2 in]
                    n106 = call-poly <vilib>:"Mean.vi"("X"=w195) -> ("mean"=w199:dbl)  [unwired: 1 out]
                    n107 = local write "element"(w199) -> ()
                    n108 = local read "Reinitialize"() -> (w209:bool)
                    n109 = local read "Automatic"() -> (w210:bool)
                    n110 = local read "Autotune"() -> (w211:bool)
                    n111 = local read "Replace Gain"() -> (w202:bool)
                    n112 = local read "MV:"() -> (w208:dbl)
                    n113 = local read "Insert Gain"() -> (w205:bool)
                    n114 = local read "autotuning parameters"() -> (w200:T4)
                    n115 = call "nonlinearcancellationVolFlow.vi"("input variable"=w199) -> ("MVT Process Variable"=w207:dbl)  [unwired: 10 in]
                    n116 = call "PID Controller_Autotuning.vi"("autotuning parameters"=w200, "PID gains in"=w203, "process variable"=w207, "dt (s)"=w198, "setpoint"=w204, "manipulated variable"=w208, "Reinitialize"=w209, "Automatic"=w210, "Autotune"=w211) -> ("Tuned PID gains"=w201:T3, "output"=w215:dbl)  [unwired: 1 in]
                    n117 = local write "PID gains out"(w203) -> ()
                    n118 = local write "MV:"(w215) -> ()
                    n119 = call-poly <vilib>:"PID.vi"("dt (s)"=w198, "PID gains"=w203, "process variable"=w207, "setpoint"=w204) -> ()  [unwired: 6 in, 2 out]
                    n120 = call <vilib>:"Boolean Crossing PtByPt.vi"("direction"=enum16{"either", "false-true", "true-false"}."false-true", "input"=w205) -> ("crossing"=w220:bool)  [unwired: 1 in]
                    n121 = call <vilib>:"Boolean Crossing PtByPt.vi"("direction"=enum16{"either", "false-true", "true-false"}."false-true", "input"=w202) -> ("crossing"=w218:bool)  [unwired: 1 in]
                    n122 = local write "MVT Process variable"(w207) -> ()
                    n123 = local write "tuned PID gains"(w201) -> ()
                    n124 = case shown="True" w220 {
                      tunnel: w217 -> [_ w243]
                      tunnel: w212 -> [_ w241]
                      tunnel: w204 -> [_ w240]
                      tunnel: w201 -> [_ w239]
                      frame False {
                      }
                      frame True {
                        n125 = Bundle("Tuned PID gains"=w239, "MVT Process Variable"=w240) -> (w238:T7)  [unwired: 1 in]
                        n126 = Increment(x=w243) -> (x+1=w242:i32)
                        n127 = Insert Into Array(array=w241, index=w242, new element=w238) -> (w237:T1)
                        n128 = local write "Gain Schedule"(w237) -> ()
                      }
                    }
                    n129 = case shown="True" w218 {
                      tunnel: w217 -> [_ w234]
                      tunnel: w212 -> [_ w233]
                      tunnel: w201 -> [_ w232]
                      frame False {
                      }
                      frame True {
                        n130 = Index Array(array=w233, index=w234) -> (element=w236:T6)
                        n131 = Unbundle(w236) -> ("max value"=w235:dbl)  [unwired: 1 out]
                        n132 = Bundle("Tuned PID gains"=w232, "max value"=w235) -> (w231:T8)  [unwired: 1 in]
                        n133 = Replace Array Subset(array=w233, new element=w231, index=w234) -> (w230:T1)
                        n134 = local write "Gain Schedule"(w230) -> ()
                      }
                    }
                    n135 = local write "Output"(w215) -> ()
                    n136 = Build Array(w215) -> (w193:dbl[])
                    n137 = local write "Channel Array"(w193) -> ()
                    n138 = local write "output"(w215) -> ()
                  }
                }
                n139 = global read "STOP_GLOBAL.vi" "ALL STOP"() -> (w143:bool)
              }
              n140 = local write "Gain Schedule"(T1 [{"PID gains"={"Kc"=2.1, "Ti"=0.05, "Td"=0.0}, "max value"=0.0}, {"PID gains"={"Kc"=0.3, "Ti"=0.08, "Td"=0.0}, "max value"=200.0}]) -> ()
              n141 = local write "Pressure Scheduling"(T1 [{"PID gains"={"Kc"=2.1, "Ti"=30.0, "Td"=3.5655}, "max value"=500.0}, {"PID gains"={"Kc"=2.1, "Ti"=30.0, "Td"=3.5655}, "max value"=850.0}]) -> ()
              n142 = Bundle(w115, w107) -> (w116:cluster{dbl[], dbl[]})  [unwired: 1 in]
              n143 = Bundle(w115, w108) -> (w113:cluster{dbl[], dbl[]})  [unwired: 1 in]
              n144 = Build Array(w113, w116) -> (→"Process Variable vs Setpoint":cluster{dbl[], dbl[]}[])
              n145 = call-poly <vilib>:"PID Lead-Lag.vi"() -> ()  [unwired: 8 in, 2 out]
              n146 = while {
                stop <- w124 stop-if-true
                # "Max Voltage"
                n147 = local read "Channel Array"() -> (w127:dbl[])
                n148 = call "OnDemand_VoltageOutput.vi"("Channel Array"=w127, "minimum voltage"=0.0, "maximum voltage"=5.067, "physical channels"="cDAQ9189-21D2231Mod6/ao0") -> ("error out"=→"error out":errorcluster)  [unwired: 5 in, 2 out]
                n149 = global read "STOP_GLOBAL.vi" "ALL STOP"() -> (w124:bool)
              }
              n150 = while {
                stop <- w123 stop-if-true
                # "Max Voltage"
                n151 = call "OnDemand_VoltageOutput.vi"("Channel Array"="Needle Valve Control", "minimum voltage"=0.0, "maximum voltage"=10.0, "physical channels"="cDAQ9189-21D2231Mod6/ao1") -> ("error out"=→"error out 4":errorcluster)  [unwired: 5 in, 2 out]
                n152 = global read "STOP_GLOBAL.vi" "ALL STOP"() -> (w123:bool)
              }
            }
            frame "Step Input" {
              # "Will wait 3 seconds to start, change in step every second"
              n153 = case shown="True" "PRESS TO START" {
                frame False {
                  # "Max Voltage"
                  n154 = call "OnDemand_VoltageOutput.vi"("Channel Array"=dbl[] [0.0], "minimum voltage"=0.0, "maximum voltage"=5.067, "physical channels"="cDAQ9189-21D2231Mod6/ao0") -> ()  [unwired: 5 in, 3 out]
                }
                frame True {
                  n155 = stacked-sequence {
                    seq-local: [_ _ _ _ _ w296 _ _ _] -> [_ _ _ _ _ _ w306 _ _]
                    seq-local: [_ _ _ _ _ _ w305 _ _] -> [_ _ _ _ _ _ _ w315 _]
                    seq-local: [w253 _ _ _ _ _ _ _ _] -> [_ w259 _ _ _ _ _ _ _]
                    seq-local: [_ w258 _ _ _ _ _ _ _] -> [_ _ _ w276 _ _ _ _ _]
                    seq-local: [_ _ _ w275 _ _ _ _ _] -> [_ _ _ _ w286 _ _ _ _]
                    seq-local: [_ _ _ _ w285 _ _ _ _] -> [_ _ _ _ _ w295 _ _ _]
                    frame #0 {
                      w253 = dbl[] [0.0]
                      # "Rest state for 3 sec"
                      # "Max Voltage"
                      n156 = call "OnDemand_VoltageOutput.vi"("Channel Array"=w253, "minimum voltage"=0.0, "maximum voltage"=5.067, "physical channels"="cDAQ9189-21D2231Mod6/ao0") -> ()  [unwired: 5 in, 3 out]
                      n157 = Wait (ms)(milliseconds to wait=u32 3000) -> ()  [unwired: 1 out]
                    }
                    frame #1 {
                      w260 = 6
                      n158 = for {
                        N: w260 -> [_]
                        shift-right: [w261] -> w258
                        shift-left: w259 -> [w268]
                        tunnel: w260 -> [w262]
                        # "Max Voltage"
                        n159 = Divide(x=5.067, y=w262) -> (x/y=w264:dbl)
                        n160 = Add(x=w268, y=w264) -> (x+y=w261:dbl[])
                        "Steps on Servo" <- w261
                        n161 = Wait (ms)(milliseconds to wait=u32 500) -> ()  [unwired: 1 out]
                        n162 = call "OnDemand_VoltageOutput.vi"("Channel Array"=w261, "minimum voltage"=0.0, "maximum voltage"=5.067, "physical channels"="cDAQ9189-21D2231Mod6/ao0") -> ()  [unwired: 5 in, 3 out]
                      }
                    }
                    frame #2 {
                      # "Max Voltage"
                      n163 = call "OnDemand_VoltageOutput.vi"("Channel Array"=dbl[] [5.067], "minimum voltage"=0.0, "maximum voltage"=5.067, "physical channels"="cDAQ9189-21D2231Mod6/ao0") -> ()  [unwired: 5 in, 3 out]
                      n164 = Wait (ms)(milliseconds to wait=u32 4000) -> ()  [unwired: 1 out]
                    }
                    frame #3 {
                      w277 = 6
                      n165 = for {
                        N: w277 -> [_]
                        shift-right: [w278] -> w275
                        shift-left: w276 -> [w284]
                        tunnel: w277 -> [_]
                        # "Max Voltage"
                        # "Until it reaches 2.067"
                        # "Reduce in steps of 0.5"
                        n166 = Subtract(x=w284, y=0.5) -> (x-y=w278:dbl[])
                        n167 = local write "Steps on Servo"(w278) -> ()
                        n168 = Wait (ms)(milliseconds to wait=u32 500) -> ()  [unwired: 1 out]
                        n169 = call "OnDemand_VoltageOutput.vi"("Channel Array"=w278, "minimum voltage"=0.0, "maximum voltage"=5.067, "physical channels"="cDAQ9189-21D2231Mod6/ao0") -> ()  [unwired: 5 in, 3 out]
                      }
                    }
                    frame #4 {
                      w287 = 6
                      n170 = for {
                        N: w287 -> [_]
                        shift-right: [w288] -> w285
                        shift-left: w286 -> [w294]
                        tunnel: w287 -> [_]
                        # "Max Voltage"
                        # "Until it reaches 2.067"
                        # "Increase in steps of 0.5"
                        n171 = Add(x=w294, y=0.5) -> (x+y=w288:dbl[])
                        n172 = local write "Steps on Servo"(w288) -> ()
                        n173 = Wait (ms)(milliseconds to wait=u32 500) -> ()  [unwired: 1 out]
                        n174 = call "OnDemand_VoltageOutput.vi"("Channel Array"=w288, "minimum voltage"=0.0, "maximum voltage"=5.067, "physical channels"="cDAQ9189-21D2231Mod6/ao0") -> ()  [unwired: 5 in, 3 out]
                      }
                    }
                    frame #5 {
                      w297 = 6
                      n175 = for {
                        N: w297 -> [_]
                        shift-right: [w298] -> w296
                        shift-left: w295 -> [w304]
                        tunnel: w297 -> [_]
                        # "Max Voltage"
                        # "Until it reaches 2.067"
                        # "Reduce in steps of 0.5"
                        n176 = Subtract(x=w304, y=0.5) -> (x-y=w298:dbl[])
                        n177 = local write "Steps on Servo"(w298) -> ()
                        n178 = Wait (ms)(milliseconds to wait=u32 500) -> ()  [unwired: 1 out]
                        n179 = call "OnDemand_VoltageOutput.vi"("Channel Array"=w298, "minimum voltage"=0.0, "maximum voltage"=5.067, "physical channels"="cDAQ9189-21D2231Mod6/ao0") -> ()  [unwired: 5 in, 3 out]
                      }
                    }
                    frame #6 {
                      n180 = for {
                        N: 6 -> [_]
                        shift-right: [w308] -> w305
                        shift-left: w306 -> [w314]
                        # "Max Voltage"
                        # "Until it reaches 2.067"
                        # "Increase in steps of 0.5"
                        n181 = Add(x=w314, y=0.5) -> (x+y=w308:dbl[])
                        n182 = local write "Steps on Servo"(w308) -> ()
                        n183 = Wait (ms)(milliseconds to wait=u32 500) -> ()  [unwired: 1 out]
                        n184 = call "OnDemand_VoltageOutput.vi"("Channel Array"=w308, "minimum voltage"=0.0, "maximum voltage"=5.067, "physical channels"="cDAQ9189-21D2231Mod6/ao0") -> ()  [unwired: 5 in, 3 out]
                      }
                    }
                    frame #7 {
                      w316 = 6
                      n185 = for {
                        N: w316 -> [_]
                        shift-right: [w317] -> _
                        shift-left: w315 -> [w323]
                        tunnel: w316 -> [_]
                        # "Max Voltage"
                        # "Until it reaches 2.067"
                        # "reduce in steps of 0.5"
                        n186 = Subtract(x=w323, y=0.5) -> (x-y=w317:dbl[])
                        n187 = local write "Steps on Servo"(w317) -> ()
                        n188 = Wait (ms)(milliseconds to wait=u32 500) -> ()  [unwired: 1 out]
                        n189 = call "OnDemand_VoltageOutput.vi"("Channel Array"=w317, "minimum voltage"=0.0, "maximum voltage"=5.067, "physical channels"="cDAQ9189-21D2231Mod6/ao0") -> ()  [unwired: 5 in, 3 out]
                      }
                    }
                    frame #8 {
                      w324 = dbl[] [0.0]
                      # "Reset to 0"
                      # "Max Voltage"
                      n190 = call "OnDemand_VoltageOutput.vi"("Channel Array"=w324, "minimum voltage"=0.0, "maximum voltage"=5.0, "physical channels"="cDAQ9189-21D2231Mod6/ao0") -> ()  [unwired: 5 in, 3 out]
                      n191 = local write "Steps on Servo"(w324) -> ()
                    }
                  }
                  n192 = while {
                    stop <- w252 stop-if-true
                    n193 = call "Elapsed Time2"() -> ("Elapsed Time (s)"=w250:dbl)  [unwired: 12 in, 7 out]
                    "Elapsed Time (s) 2" <- w250
                    n194 = global read "STOP_GLOBAL.vi" "ALL STOP"() -> (w252:bool)
                    n195 = Greater?(x=w250, y=3.0 ("x")) -> (0:→"HAS 3 SECONDS PASSED?":bool)
                  }
                }
              }
            }
            frame "Do nothing" {
            }
          }
          n196 = call <vilib>:"High Resolution Relative Seconds.vi"() -> ("relative seconds"=w64:dbl)
          n197 = while {
            tunnel: "Types of Testing" -> [w379]
            tunnel: [w405] -> w77 mode=indexing
            shift-right: [w399] -> w57
            shift-left: w61 -> [w401]
            shift-right: [w380] -> w58
            shift-left: w62 -> [w400]
            tunnel: [w389] -> w78 mode=indexing
            tunnel: [w387] -> w74 mode=indexing
            tunnel: [w386] -> w79 mode=indexing
            tunnel: [w385] -> w80 mode=indexing
            tunnel: [w381] -> w66 mode=indexing
            tunnel: [w369] -> w73 mode=indexing
            tunnel: [w388] -> w72 mode=indexing
            tunnel: w64 -> [w372]
            tunnel: w63 -> [_]
            tunnel: w59 -> [w368]
            stop <- w366 stop-if-true
            w358 = 110.0 ("x")
            w403 = 10.0  # timeout (s)
            # "Add SetPoint History\nAdd Gain history to data"
            # "First Test:\n2.1\n70\n3.566\nSecond:\n2.1\n80\n3.566\nThird:\n3.1\n60\n3.566\nFourth:\n10.1\n70\n3.566"
            # "Supply\nSecond Transducer\nFlow\nTemp\nOutput Voltage"
            # "4 NI 9219 Channels"
            # "Data Collection"
            n198 = call <vilib>:"High Resolution Relative Seconds.vi"() -> ("relative seconds"=w373:dbl)
            n199 = Subtract(x=w373, y=w372) -> (x-y=w370:dbl)
            n200 = Subtract(x=w370, y=0.0) -> (x-y=w369:dbl)
            "Entire Runtime" <- w369
            n201 = call-poly <vilib>:"DAQmx Read.vi"("task/channels in"=w400, "number of samples per channel"=30, "timeout"=w403, "error in"=w401) -> ("task out"=w380:refnum<k21>, "data"=w349:waveform(dbl)[], "error out"=w399:errorcluster)  [unwired: 9 in]
            n202 = local read "PID gains out"() -> (w365:T3)
            n203 = local read "Actual Clock Rate"() -> (w375:dbl)
            n204 = global read "STOP_GLOBAL.vi" "ALL STOP"() -> (w402:bool)
            n205 = Unbundle By Name(w399) -> ("status"=w404:bool)
            n206 = Split Signals(w349) -> (w348:dynamicdata, w347:dynamicdata, w346:dynamicdata, w345:dynamicdata, w344:dynamicdata, w343:dynamicdata, w342:dynamicdata, w341:dynamicdata, w340:dynamicdata, w339:dynamicdata, w338:dynamicdata, w337:dynamicdata)  [unwired: 13 in, 1 out]
            n207 = Unbundle By Name(w365) -> ("proportional gain (Kc)"=w361:dbl, "integral time (Ti, min)"=w362:dbl, "derivative time (Td, min)"=w363:dbl)
            n208 = Divide(x=1.0, y=w375) -> (x/y=w374:dbl)
            n209 = local read "SP"() -> (w364:dbl)
            n210 = Or(x=w404, y=w402) -> (x .or. y?=w366:bool)
            n211 = Multiply(x=1000.0, y=w374) -> (x*y=w367:dbl)
            n212 = Merge Signals(w348, w347, w346, w345, w344, w343, w342, w341, w340, w339, w338, w337) -> (w398:dynamicdata)
            n213 = Wait Until Next ms Multiple(millisecond multiple=w367) -> ()  [unwired: 1 out]
            n214 = call "Filter3"("Signal"=w398) -> ("Filtered Signal"=w336:dynamicdata)  [unwired: 9 in, 1 out]
            n215 = call "Convert to Dynamic Data2"("Double"=w361) -> ("Dynamic Data Type"=w353:dynamicdata)  [unwired: 3 in]
            n216 = call "Convert to Dynamic Data3"("Double"=w362) -> ("Dynamic Data Type"=w354:dynamicdata)  [unwired: 3 in]
            n217 = call "Convert to Dynamic Data4"("Double"=w363) -> ("Dynamic Data Type"=w355:dynamicdata)  [unwired: 3 in]
            n218 = call "Convert to Dynamic Data"("Double"=w364) -> ("Dynamic Data Type"=w356:dynamicdata)  [unwired: 3 in]
            n219 = Split Signals(w336) -> (w335:dynamicdata, w334:dynamicdata, w333:dynamicdata, w332:dynamicdata, w331:dynamicdata, w330:dynamicdata, w329:dynamicdata, w328:dynamicdata)  [unwired: 13 in, 5 out]
            n220 = local write "Temperature"(w328) -> ()
            n221 = Merge Signals(w335, w334, w331, w328, w330, w353, w354, w355, w356) -> (w360:dynamicdata)
            n222 = Multiply(x=w330, y=18.0) -> (x*y=w351:dynamicdata)
            n223 = local write "Voltage Output"(w351) -> ()
            n224 = Multiply(x=w358, y=w335) -> (x*y=w359:dynamicdata)
            n225 = Multiply(x=w358, y=w334) -> (x*y=w394:dynamicdata)
            n226 = Multiply(x=w358, y=w332) -> (x*y=w393:dynamicdata)
            n227 = Multiply(x=200.0, y=w331) -> (x*y=w391:dynamicdata)
            n228 = Multiply(x=w358, y=w333) -> (x*y=w357:dynamicdata)
            n229 = Merge Signals(w335, w334, w332, w331, w333, w329, w328, w330, w353, w354, w355, w356) -> (w378:dynamicdata)
            n230 = call "Convert from Dynamic Data11"("Dynamic Data Type"=w394) -> ("Array"=w395:dbl[])  [unwired: 3 in]
            n231 = call "Convert from Dynamic Data8"("Dynamic Data Type"=w359) -> ("Array"=w396:dbl[])  [unwired: 3 in]
            n232 = call "Convert from Dynamic Data12"("Dynamic Data Type"=w393) -> ("Array"=w392:dbl[])  [unwired: 3 in]
            n233 = call "Convert from Dynamic Data13"("Dynamic Data Type"=w391) -> ("Array"=w390:dbl[])  [unwired: 3 in]
            n234 = local write "Inlet Pressure"(w357) -> ()
            n235 = call-poly <vilib>:"Mean.vi"("X"=w396) -> ("mean"=w389:dbl)  [unwired: 1 out]
            n236 = call-poly <vilib>:"Mean.vi"("X"=w395) -> ("mean"=w388:dbl)  [unwired: 1 out]
            n237 = call-poly <vilib>:"Mean.vi"("X"=w392) -> ("mean"=w387:dbl)  [unwired: 1 out]
            n238 = call-poly <vilib>:"Mean.vi"("X"=w390) -> ("mean"=w386:dbl)  [unwired: 1 out]
            n239 = case shown="\"Test Firing\", Default" w379 {
              tunnel: w360 -> [_ w440]
              tunnel: w378 -> [w419 _]
              tunnel: w368 -> [w414 w431]
              frame "Test Firing", Default {
                n240 = Build Array("Supply Pressure", "Second Pressure Transducer", "Chamber Pressure", "Volumetric Flow", "Inlet Pressure", "Thrust", "Temperature", "Voltage Out" ("element"), "Kc" ("element"), "Ti" ("element"), "Td" ("element"), "Setpoint" ("element")) -> (w417:string[])
                n241 = call "RenameDynamicSignals.vi"("New Signal Names"=w417, "Dynamic Data In"=w419) -> ("error out"=w415:errorcluster, "Dynamic Data Out"=w416:dynamicdata)  [unwired: 2 in]
                n242 = call "Write To Measurement File3"("Signals"=w416, "Enable"="Collect Data?", "error in (no error)"=w415, "Filename"=w414) -> ("Filename Out"=→"Filename Out":path, "Saving Data"=→"Saving Data":bool, "error out"=→"error out 3":errorcluster)  [unwired: 13 in]
              }
              frame "Cold Flow Rig" {
                n243 = Build Array("Supply Pressure", "Second Pressure Transducer", "Volumetric Flow", "Temperature", "Voltage Out" ("element"), "Kc" ("element"), "Ti" ("element"), "Td" ("element"), "Setpoint" ("element")) -> (w434:string[])
                n244 = call "RenameDynamicSignals.vi"("New Signal Names"=w434, "Dynamic Data In"=w440) -> ("error out"=w432:errorcluster, "Dynamic Data Out"=w433:dynamicdata)  [unwired: 2 in]
                n245 = call "Write To Measurement File4"("Signals"=w433, "Enable"="Collect Data? 2", "error in (no error)"=w432, "Filename"=w431) -> ("Filename Out"=→"Filename Out":path, "Saving Data"=→"Saving Data":bool)  [unwired: 13 in, 1 out]
              }
            }
            n246 = local write "Supply Pressure PSI"(w359) -> ()
            n247 = local write "Thrust lb"(w329) -> ()
            n248 = local write "Chamber Pressure PSI"(w393) -> ()
            n249 = local write "Vol Flow L/min"(w391) -> ()
            n250 = local write "Line Pressure"(w394) -> ()
            n251 = call "Convert from Dynamic Data3"("Dynamic Data Type"=w328) -> ("Array"=w383:dbl[])  [unwired: 3 in]
            n252 = call "Convert from Dynamic Data4"("Dynamic Data Type"=w351) -> ("Array"=w382:dbl[])  [unwired: 3 in]
            n253 = call "Convert from Dynamic Data"("Dynamic Data Type"=w329) -> ("Array"=w384:dbl[])  [unwired: 3 in]
            n254 = call-poly <vilib>:"Mean.vi"("X"=w382) -> ("mean"=w381:dbl)  [unwired: 1 out]
            n255 = call-poly <vilib>:"Mean.vi"("X"=w384) -> ("mean"=w405:dbl)  [unwired: 1 out]
            n256 = call-poly <vilib>:"Mean.vi"("X"=w383) -> ("mean"=w385:dbl)  [unwired: 1 out]
          }
          n257 = call <vilib>:"DAQmx Stop Task.vi"("task/channels in"=w58, "error in"=w57) -> ("task out"=w55:refnum<k21>, "error out"=w56:errorcluster)  [unwired: 12 in]
          n258 = call <vilib>:"DAQmx Clear Task.vi"("task in"=w55, "error in"=w56) -> ("error out"=w54:errorcluster)  [unwired: 13 in]
          "error out 2" <- w54
          n259 = Bundle(w73, w72) -> (w71:cluster{dbl[], dbl[]})  [unwired: 1 in]
          "Second Pressure Transducer" <- w71
          n260 = Bundle(w73, w74) -> (w70:cluster{dbl[], dbl[]})  [unwired: 1 in]
          "Chamber Pressure" <- w70
          n261 = Bundle(w73, w78) -> (w76:cluster{dbl[], dbl[]})  [unwired: 1 in]
          "Supply Pressure" <- w76
          n262 = Bundle(w73, w79) -> (w69:cluster{dbl[], dbl[]})  [unwired: 1 in]
          "MassFlow" <- w69
          n263 = Bundle(w73, w77) -> (w68:cluster{dbl[], dbl[]})  [unwired: 1 in]
          "Thrust" <- w68
          n264 = Bundle(w73, w80) -> (w67:cluster{dbl[], dbl[]})  [unwired: 1 in]
          "Temperature" <- w67
          n265 = Bundle(w73, w66) -> (→"Servo Voltage Output":cluster{dbl[], dbl[]})  [unwired: 1 in]
          n266 = call <vilib>:"Simple Error Handler.vi"("error in (no error)"=w54) -> ()  [unwired: 4 in, 5 out]
          n267 = Build Array(w76, w71, w70, w69, w68, w67) -> (→"All Channel Graph":cluster{dbl[], dbl[]}[])
        }
      }
    }
  }
